vi "demo.vi"() -> ()   [LabVIEW 2014]
uses:
  Instance           7 12Saved   demo .vi
  Instance           3 12Saved   demo .vi
  Instance           6 12Saved   demo .vi
  Instance           4 12Saved   demo .vi
  Instance           5 12Saved   demo .vi
  Instance           2 12Saved   demo .vi
  Instance           1 12Saved   demo .vi
  ControlCAN.dll
panel:
  out "retok1":bool
  out "retok0":bool
  in  "Radio_Baud 2":bool=TRUE
  in  "e-u-baud 2":cluster{"数值":u32}
  out "VCI_INIT_CONFIG 2":T1={"AccCode"=0, "AccMask"=4294967295, "Reserved"=0, "Filter"=1, "Timing0"=0, "Timing1"=20, "Mode"=0}
  in  "?":enum32{"选项卡 1"}(tab)
  out "VF控制频率":dbl caption="Beta"
  out "母线电流":dbl caption="Beta"
  in  "扭矩梯度":dbl caption="Beta"
  in  "打开曲线":bool
  in  "CAN通道0":u32 caption="CAN"
  in  "StartCAN":bool
  in  "设备类型":u32(ring)=1 items=["PCI5121"=1, "PCI9810"=2, "USBCAN1"=3, "USBCAN2"=4, "PCI9820"=5, "PCI5110"=7, "PC104CAN"=11, "CANETUDP"=12, "PCI9840B"=14, "PC104C2"=15, "PCI9820I"=16, "CANETTCP"=17, "PCIE9221"=24, "PCI5010U"=19, "USBCAN_E_U"=20, "USBCAN_2E_U"=21, "PCI5020U"=22, "PCIE9120I"=27, "PCIE9110I"=28, "PCIE9140I"=29]
  in  "OpenDevice":bool
  in  "DeviceOpen":bool
  out "CANStartup":bool
  in  "Baud":u32(ring)=11 caption="波特率" items=["5Kbps", "10Kbps", "20Kbps", "40Kbps", "50Kbps", "80Kbps", "100Kbps", "125Kbps", "200Kbps", "250Kbps", "400Kbps", "500Kbps", "666Kbps", "800Kbps", "1000Kbps"]
  in  "索引":u32(ring) items=["0", "1", "2", "3", "4", "5", "6", "7", "8"]
  out "电位器值":i16 caption="Beta"
  out "母线电流零漂":u16 caption="Beta"
  out "V相电流":dbl
  in  "保存路径 2":path caption="保存路径"
  out "记录计数 3":u32 caption="已记录"
  in  "自动记录 2":bool
  out "U电流零漂":u16 caption="Beta"
  out "V电流零漂":u16 caption="Beta"
  out "U相电流":dbl caption="Beta"
  out "W相电流":dbl caption="Beta"
  in  "控制模式":u8(ring) items=["停车", "速度控制", "扭矩控制"]
  out "母线电压":dbl caption="Beta"
  out "电角度":u16
  out "D轴电压Vd":dbl
  out "Q轴电压Vq":dbl caption="Beta"
  out "Id电流":dbl caption="Beta"
  out "Iq电流":dbl caption="Beta"
  out "Id电流指令":dbl
  out "Iq电流指令":dbl caption="Beta"
  out "控制模式":u8(ring) items=["停车", "速度控制", "扭矩控制", "VqVF控制", "VdVq控制", "IdIq控制"]
  out "相电流Is":dbl caption="Beta"
  out "相电压Vs":dbl caption="Beta"
  in  "确定发送":bool
  in  "转矩指令":dbl caption="Beta"
  out "电机扭矩":dbl caption="Beta"
  in  "转速梯度":dbl caption="Beta"
  in  "增加":bool
  in  "减少":bool
  in  "增加 2":bool
  in  "减少 2":bool
  in  "故障恢复":bool
  out "系统报警码":u16 caption="Beta"
  out "波形图表":T2(graph)
  in  "给定转速":dbl caption="Beta"
  out "电机转速":dbl caption="Beta"
  in  "选项卡控件":enum32{"选项卡 1"}(tab)
  in  "TREvent":T3={"Tx_Or_Rx"=FALSE, "VCI_CAN_OBJ"={"ID"=0, "TimeStamp"=0, "TimeFlag"=0, "SendType"=1, "RemoteFlag"=0, "ExternFlag"=0, "DataLen"=8, 0, 0, 0, 0, 0, 0, 0, 0, 0, 0, 0}, "VCI_CAN_OBJ_N"=[], "Num"=0}
  in  "滤波模式":u32(ring) items=["标准帧滤波", "扩展帧滤波", "禁能滤波"]
  in  "寄存器":u32 format="0x%08x"
  in  "Radio_Baud(E_U)":bool=TRUE
  in  "CANET IP":string
  in  "stop":bool
  in  "发送类型":u8(ring) items=["正常发送", "单次发送", "自发自收", "单次自发自收"]
  in  "帧类型":u8(ring) items=["标准帧", "扩展帧"]
  in  "帧格式":u8(ring) items=["数据帧", "远程帧"]
  in  "数据输入":string
  in  "ID":u32 format="0x%08x"
  in  "验收码":u32 format="0x%08x"
  in  "屏蔽码":u32=4294967295 format="0x%08x"
  in  "BTR0":u8 format="0x%02x"
  in  "BTR1":u8=20 format="0x%02x"
  in  "滤波方式":u8(ring) items=["双滤波", "单滤波"]
  in  "模式":u8(ring) items=["正常", "只听"]
  in  "Clear Buffer":bool
  in  "GetBoardInfo":bool
  in  "GetErrorInfo":bool
  in  "GetStatus":bool
  in  "SEND_NCAN":bool
  in  "滤波结束ID":u32
  in  "滤波起始ID":u32
  in  "一次发送帧数":u32
  in  "Radio_Baud":bool=TRUE
  in  "BTR1 2":u8=20 format="0x%02x"
  in  "BTR0 2":u8 format="0x%02x"
  in  "寄存器 2":u32 format="0x%08x"
  in  "确定发送 2":bool
  in  "ResetCAN":bool
  out "CANStartup 2":bool
  in  "StartCAN 2":bool
  in  "CAN 通道 2":u32=1 caption="CAN"
  in  "Baud 2":u32(ring) caption="波特率2" items=["5Kbps", "10Kbps", "20Kbps", "40Kbps", "50Kbps", "80Kbps", "100Kbps", "125Kbps", "200Kbps", "250Kbps", "400Kbps", "500Kbps", "666Kbps", "800Kbps", "1000Kbps"]
  out "VCI_CAN_OBJ_TN":T4(array[cluster])
  out "VCI_CAN_OBJ_RN":T4(array[cluster])
  in  "arraylen":u32
  out "type":u8[](array[numeric])
  in  "本机端口":u32
  in  "本机类型":enum32{"Radio Selection 1", "Radio Selection 2"}(radio)
  in  "CANET 端口":u32
  out "VCI_FILTER_RECORD":cluster{"ExtFrame":u32, "Start":u32, "End":u32}
  in  "e-u-baud":cluster{"数值":u32}
  out "VCI_CAN_OBJ_T_N":T4(array[cluster])
  out "VCI_BOARD_INFO":T5
  out "VCI_ERR_INFO":T6
  out "VCI_CAN_STATUS":T7
  out "stop 2":bool
  out "Num Rows":u32
  out "TRCount":u32
  out "VCI_CAN_OBJ_R":T8={"ID"=0, "TimeStamp"=0, "TimeFlag"=0, "SendType"=1, "RemoteFlag"=0, "ExternFlag"=0, "DataLen"=8, 0, 0, 0, 0, 0, 0, 0, 0, 0, 0, 0}
  out "VCI_CAN_OBJ_T":T8={"ID"=0, "TimeStamp"=0, "TimeFlag"=0, "SendType"=1, "RemoteFlag"=0, "ExternFlag"=0, "DataLen"=8, 0, 0, 0, 0, 0, 0, 0, 0, 0, 0, 0}
  out "VCI_INIT_CONFIG":T1={"AccCode"=0, "AccMask"=4294967295, "Reserved"=0, "Filter"=1, "Timing0"=0, "Timing1"=20, "Mode"=0}
  # "_U系列特殊设置"
  # "CANET 设备特殊设置"
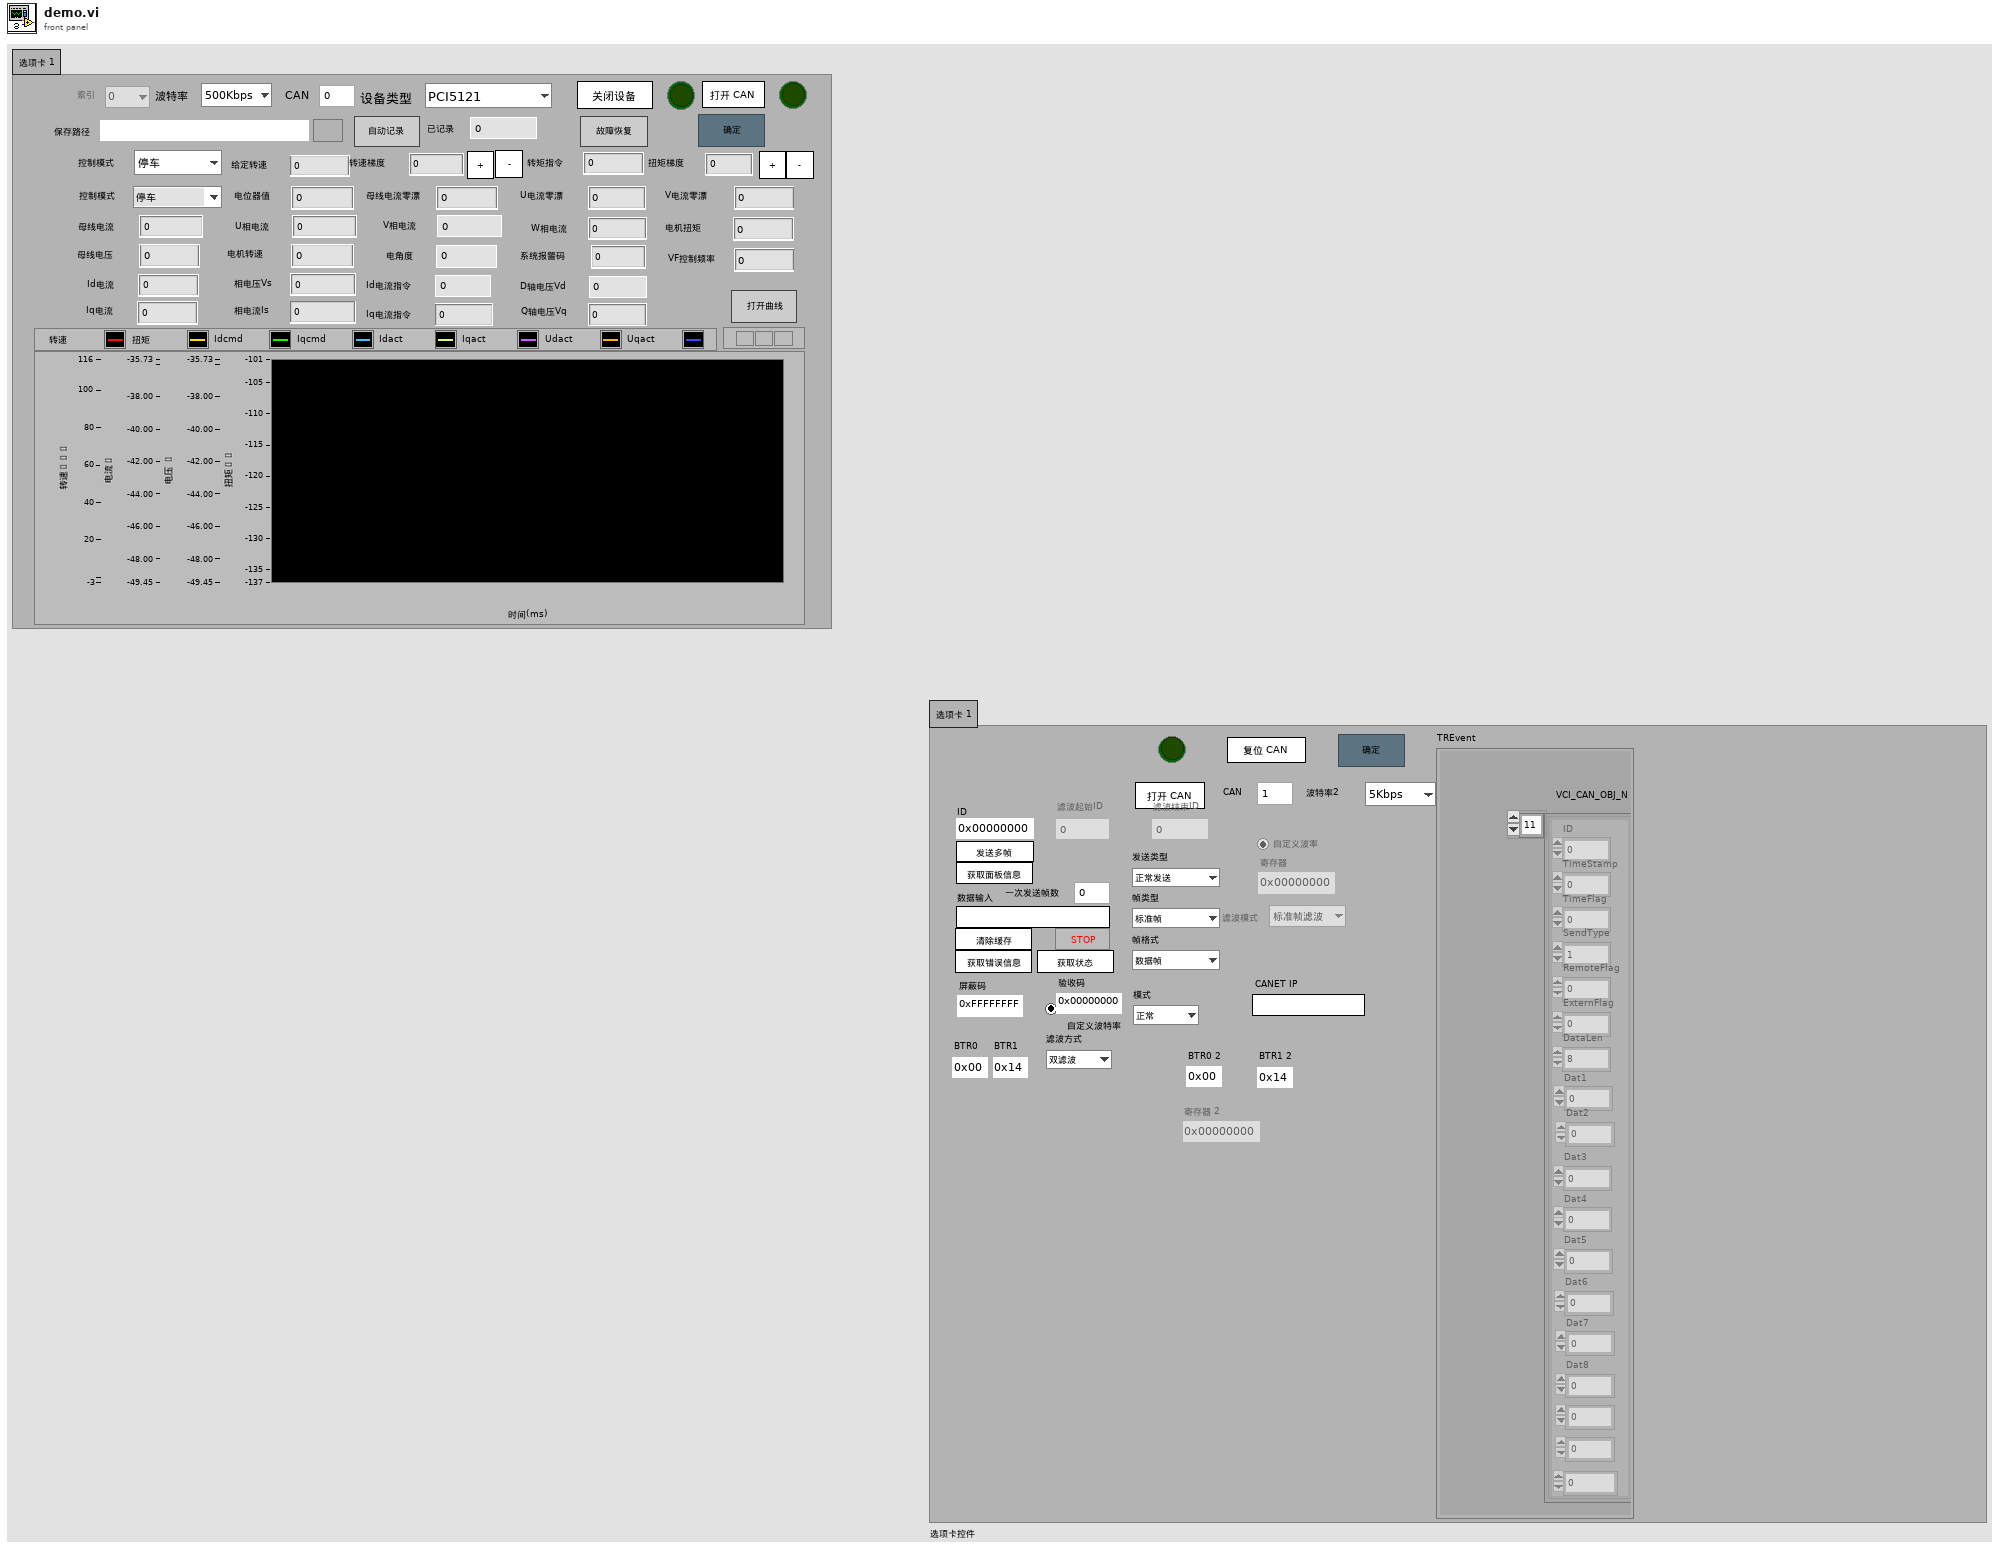
[diagram p1: front panel]
types:
  T1 = cluster{"AccCode":u32, "AccMask":u32, "Reserved":u32, "Filter":u8, "Timing0":u8, "Timing1":u8, "Mode":u8}
  T2 = cluster{"电机转速 ":dbl, " 电机扭矩":dbl, "D轴电流指令":dbl, "Q轴电流指令":dbl, "D轴电流Id":dbl, "Q轴电流Iq":dbl, "D轴电压Vd":dbl, "Q轴电压Vq":dbl}
  T3 = cluster{"Tx_Or_Rx":bool, "VCI_CAN_OBJ":cluster{"ID":u32, "TimeStamp":u32, "TimeFlag":u8, "SendType":u8, "RemoteFlag":u8, "ExternFlag":u8, "DataLen":u8, u8, u8, u8, u8, u8, u8, u8, u8, u8, u8, u8}, "VCI_CAN_OBJ_N":cluster{"ID":u32, "TimeStamp":u32, "TimeFlag":u8, "SendType":u8, "RemoteFlag":u8, "ExternFlag":u8, "DataLen":u8, "Dat1":u8, "Dat2":u8, "Dat3":u8, "Dat4":u8, "Dat5":u8, "Dat6":u8, "Dat7":u8, "Dat8":u8, u8, u8, u8}[], "Num":u32}
  T4 = cluster{"ID":u32, "TimeStamp":u32, "TimeFlag":u8, "SendType":u8, "RemoteFlag":u8, "ExternFlag":u8, "DataLen":u8, u8, u8, u8, u8, u8, u8, u8, u8, u8, u8, u8}[]
  T5 = cluster{"hw_Version":u16, "fw_Version":u16, "dr_Version":u16, "in_Version":u16, "irq_Num":u16, "can_Num":u8, "str_Serial_Num 0":i8, "str_Serial_Num 1":i8, "str_Serial_Num 2":i8, "str_Serial_Num 3":i8, "str_Serial_Num 4":i8, "str_Serial_Num 5":i8, "str_Serial_Num 6":i8, "str_Serial_Num 7":i8, "str_Serial_Num 8":i8, "str_Serial_Num 9":i8, "str_Serial_Num 10":i8, "str_Serial_Num 11":i8, "str_Serial_Num 12":i8, "str_Serial_Num 13":i8, "str_Serial_Num 14":i8, "str_Serial_Num 15":i8, "str_Serial_Num 16":i8, "str_Serial_Num 17":i8, "str_Serial_Num 18":i8, "str_Serial_Num 19":i8, "str_hw_Type 0":i8, "str_hw_Type 1":i8, "str_hw_Type 2":i8, "str_hw_Type 3":i8, "str_hw_Type 4":i8, "str_hw_Type 5":i8, "str_hw_Type 6":i8, "str_hw_Type 7":i8, "str_hw_Type 8":i8, "str_hw_Type 9":i8, "str_hw_Type 10":i8, "str_hw_Type 11":i8, "str_hw_Type 12":i8, "str_hw_Type 13":i8, "str_hw_Type 14":i8, "str_hw_Type 15":i8, "str_hw_Type 16":i8, "str_hw_Type 17":i8, "str_hw_Type 18":i8, "str_hw_Type 19":i8, "str_hw_Type 20":i8, "str_hw_Type 21":i8, "str_hw_Type 22":i8, "str_hw_Type 23":i8, "str_hw_Type 24":i8, "str_hw_Type 25":i8, "str_hw_Type 26":i8, "str_hw_Type 27":i8, "str_hw_Type 28":i8, "str_hw_Type 29":i8, "str_hw_Type 30":i8, "str_hw_Type 31":i8, "str_hw_Type 32":i8, "str_hw_Type 33":i8, "str_hw_Type 34":i8, "str_hw_Type 35":i8, "str_hw_Type 36":i8, "str_hw_Type 37":i8, "str_hw_Type 38":i8, "str_hw_Type 39":i8, "Reserved 0":u16, "Reserved 1":u16, "Reserved 2":u16, "Reserved 3":u16}
  T6 = cluster{"ErrCode":u32, "Passive_ErrData0":u8, "Passive_ErrData1":u8, "Passive_ErrData2":u8, "ArLost_ErrData":u8}
  T7 = cluster{"ErrInterrupt":u8, "regMode":u8, "regStatus":u8, "regALCapture":u8, "regECCapture":u8, "regEWLimit":u8, "regRECounter":u8, "regTECounter":u8, "Reserved":u32}
  T8 = cluster{"ID":u32, "TimeStamp":u32, "TimeFlag":u8, "SendType":u8, "RemoteFlag":u8, "ExternFlag":u8, "DataLen":u8, u8, u8, u8, u8, u8, u8, u8, u8, u8, u8, u8}
  T9 = cluster{"[0]":u32, "[1]":u32, "[2]":u32, "[3]":u32, "[4]":u32, "[5]":u32, "[6]":u32, "[7]":u32, "[8]":u32}
  T10 = cluster{"ID":u32, u32, u8, "发送类型":u8, "帧格式":u8, "帧类型":u8, i32, "[0]":u32, "[1]":u32, "[2]":u32, "[3]":u32, "[4]":u32, "[5]":u32, "[6]":u32, "[7]":u32, u8, u8, u8}
  T11 = cluster{"验收码":u32, "屏蔽码":u32, i32, "滤波方式":u8, "BTR0 2":u8, "BTR1 2":u8, "模式":u8}
  T12 = cluster{"验收码":u32, "屏蔽码":u32, u32, "滤波方式":u8, "BTR0":u8, "BTR1":u8, "模式":u8}
  T13 = cluster{"ID":u32, "TimeStamp":u32, "TimeFlag":u8, "SendType":u8, "RemoteFlag":u8, "ExternFlag":u8, "DataLen":u8, "Dat1":u8, "Dat2":u8, "Dat3":u8, "Dat4":u8, "Dat5":u8, "Dat6":u8, "Dat7":u8, "Dat8":u8, u8, u8, u8}[]
  T14 = cluster{"0x55":u32, u32, u8, "发送类型":u8, "帧格式":u8, "帧类型":u8, i32, "控制模式":u8, i16, u8, u8, u8, u8, u8, u8, u8, u8, u8}
  T15 = cluster{"0x55":u32, u32, u8, "发送类型":u8, "帧格式":u8, "帧类型":u8, i32, "控制模式":u8, u8, u8, u8, u8, u8, u8, u8, u8, u8, u8}
  T16 = cluster{bool, "VCI_CAN_OBJ_R":cluster{"ID":u32, "TimeStamp":u32, "TimeFlag":u8, "SendType":u8, "RemoteFlag":u8, "ExternFlag":u8, "DataLen":u8, u8, u8, u8, u8, u8, u8, u8, u8, u8, u8, u8}, "pReceive":cluster{"ID":u32, "TimeStamp":u32, "TimeFlag":u8, "SendType":u8, "RemoteFlag":u8, "ExternFlag":u8, "DataLen":u8, u8, u8, u8, u8, u8, u8, u8, u8, u8, u8, u8}[], "return type":u32}
  T17 = cluster{bool, "VCI_CAN_OBJ_T":cluster{"ID":u32, "TimeStamp":u32, "TimeFlag":u8, "SendType":u8, "RemoteFlag":u8, "ExternFlag":u8, "DataLen":u8, u8, u8, u8, u8, u8, u8, u8, u8, u8, u8, u8}, cluster{"ID":u32, "TimeStamp":u32, "TimeFlag":u8, "SendType":u8, "RemoteFlag":u8, "ExternFlag":u8, "DataLen":u8, u8, u8, u8, u8, u8, u8, u8, u8, u8, u8, u8}[], "return type":u32}
  T18 = cluster{"电机转速 ":dbl, " 电机扭矩":dbl, "Id电流指令":dbl, "Iq电流指令":dbl, "Id电流":dbl, "Iq电流":dbl, "D轴电压Vd":dbl, "Q轴电压Vq":dbl}
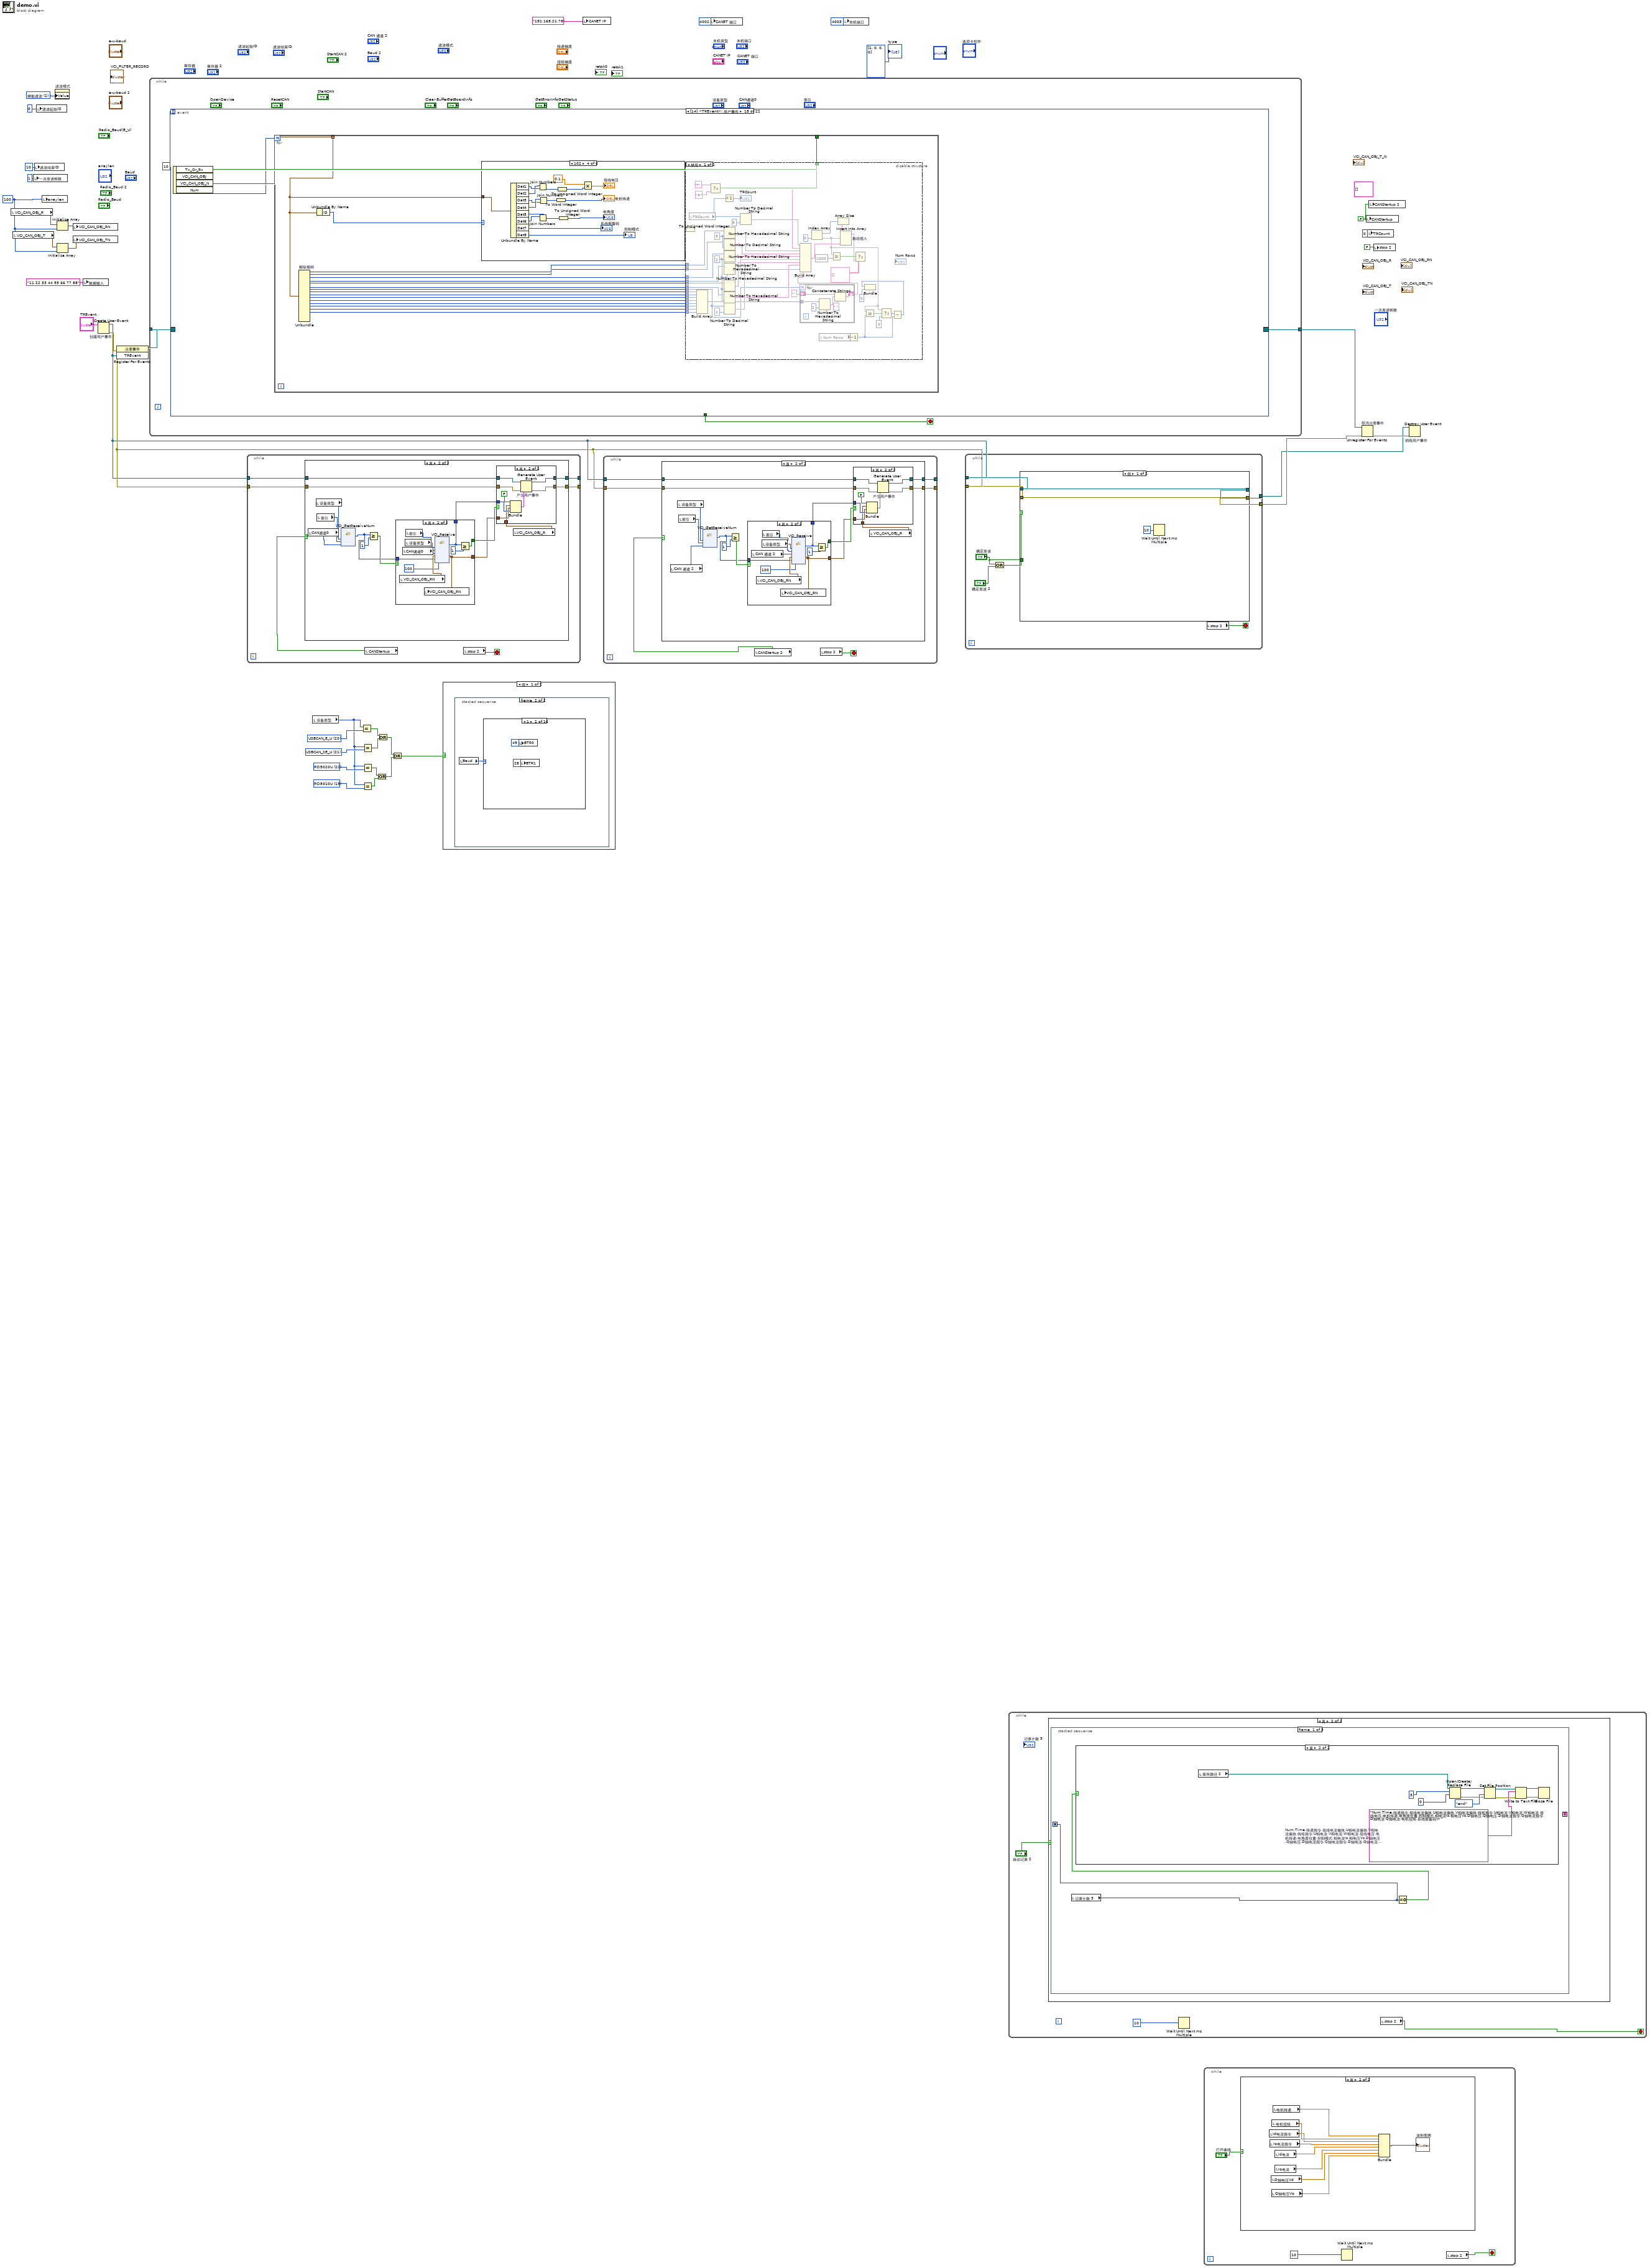
[diagram p0: block diagram]
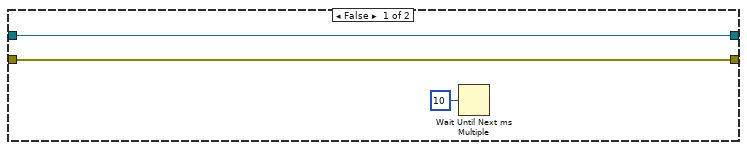
[diagram p2: hidden frame]
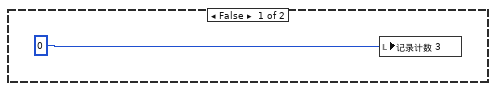
[diagram p6: hidden frame]
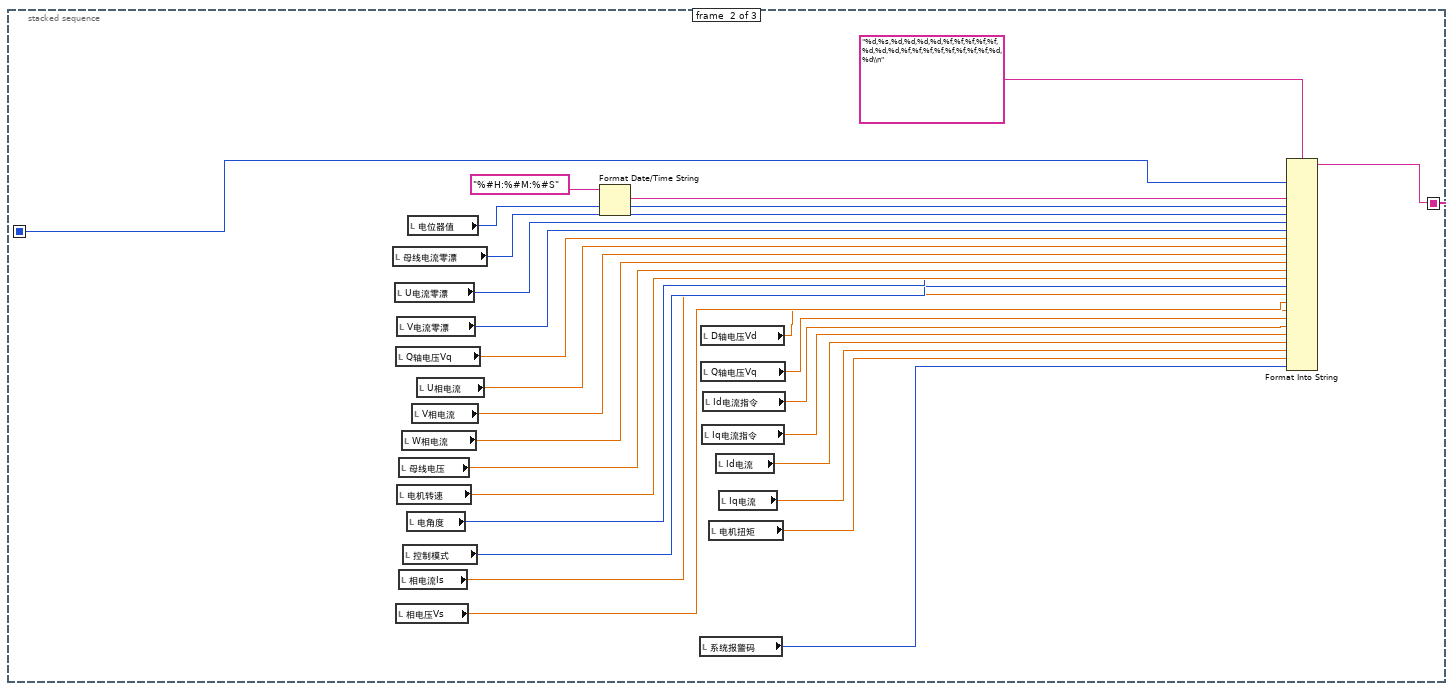
[diagram p8: hidden frame]
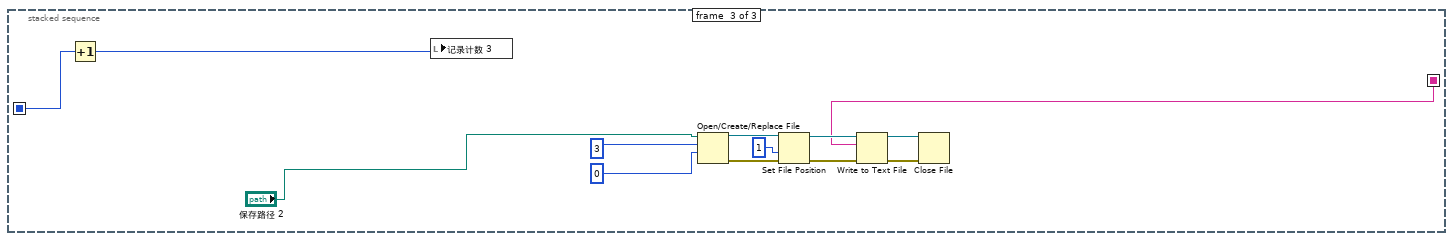
[diagram p9: hidden frame]
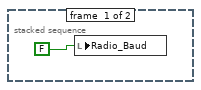
[diagram p10: hidden frame]
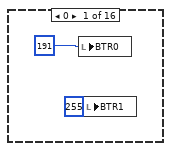
[diagram p11: hidden frame]
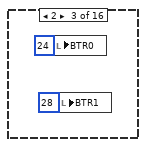
[diagram p12: hidden frame]
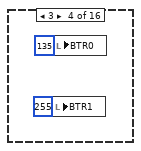
[diagram p13: hidden frame]
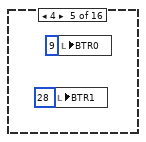
[diagram p14: hidden frame]
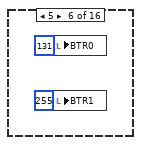
[diagram p15: hidden frame]
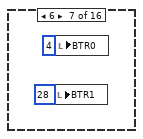
[diagram p16: hidden frame]
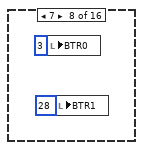
[diagram p17: hidden frame]
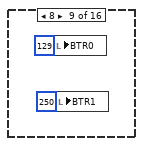
[diagram p18: hidden frame]
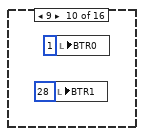
[diagram p19: hidden frame]
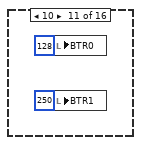
[diagram p20: hidden frame]
diagram:
  w13 = u32 19 items=["PCI5121"=1, "PCI9810"=2, "USBCAN1"=3, "USBCAN2"=4, "PCI9820"=5, "PCI5110"=7, "CANLite(mini)"=8, "ISA9620"=9, "ISA5420"=10, "PC104CAN"=11, "DNP9810"=13, "PCI9840B"=14, "PC104C2"=15, "PCI9820I"=16, "pec9920"=18, "PCI5010U"=19, "USBCAN_E_U"=20, "USBCAN_2E_U"=21, "PCI5020U"=22, ""=0] ("DeviceType")
  w14 = u32 22 items=["PCI5121"=1, "PCI9810"=2, "USBCAN1"=3, "USBCAN2"=4, "PCI9820"=5, "PCI5110"=7, "CANLite(mini)"=8, "ISA9620"=9, "ISA5420"=10, "PC104CAN"=11, "DNP9810"=13, "PCI9840B"=14, "PC104C2"=15, "PCI9820I"=16, "pec9920"=18, "PCI5010U"=19, "USBCAN_E_U"=20, "USBCAN_2E_U"=21, "PCI5020U"=22, ""=0] ("DeviceType")
  w15 = u32 21 items=["PCI5121"=1, "PCI9810"=2, "USBCAN1"=3, "USBCAN2"=4, "PCI9820"=5, "PCI5110"=7, "CANLite(mini)"=8, "ISA9620"=9, "ISA5420"=10, "PC104CAN"=11, "DNP9810"=13, "PCI9840B"=14, "PC104C2"=15, "PCI9820I"=16, "pec9920"=18, "USBCAN_E_U"=20, "USBCAN_2E_U"=21, ""=0] ("DeviceType")
  w16 = u32 20 items=["PCI5121"=1, "PCI9810"=2, "USBCAN1"=3, "USBCAN2"=4, "PCI9820"=5, "PCI5110"=7, "CANLite(mini)"=8, "ISA9620"=9, "ISA5420"=10, "PC104CAN"=11, "DNP9810"=13, "PCI9840B"=14, "PC104C2"=15, "PCI9820I"=16, "pec9920"=18, "USBCAN_E_U"=20, "USBCAN_2E_U"=21, ""=0] ("DeviceType")
  w22 = u32 100 ("arraylen")
  w30 = u32 2 items=["标准帧滤波", "扩展帧滤波", "禁能滤波"] ("fiter_mode")
  (unwired) string[][] [] ("Item Names")
  w4 = FALSE
  n1 = local read "VCI_CAN_OBJ_R"() -> (w25:T8)
  n2 = local read "VCI_CAN_OBJ_T"() -> (w23:T8)
  n3 = local write "一次发送帧数"(u32 1 ("一次发送帧数")) -> ()
  n4 = local write "滤波结束ID"(u32 10 ("fiter_endid")) -> ()
  n5 = local write "滤波起始ID"(u32 0 ("fiter_startid")) -> ()
  n6 = local write "arraylen"(w22) -> ()
  n7 = property on="滤波模式" class="Ring (严格)"("Value"=w30) -> ()  [unwired: 2 in, 2 out]
  n8 = Initialize Array(w25, w22) -> (w24:T4)
  n9 = Initialize Array(w23, w22) -> (w21:T4)
  n10 = local write "VCI_CAN_OBJ_RN"(w24) -> ()
  n11 = local write "VCI_CAN_OBJ_TN"(w21) -> ()
  n12 = local write "数据输入"("11 22 33 44 55 66 77 88" ("Data Input")) -> ()
  n13 = Create User Event "创建用户事件"(user event datatype="TREvent") -> (user event=w3:refnum<user-event>, error out=w37:errorcluster)  [unwired: 1 in]
  n14 = register-events(error in=w37, w3) -> (reference out=w34:refnum<event-registration>, error out=w2:errorcluster)  [unwired: 1 in]
  n15 = while {
    tunnel: w34 -> [w42]
    tunnel: [w41] -> w1
    stop <- w39 stop-if-true
    n16 = event shown="[14] <TREvent>: 用户事件" {
      selector: w42 -> [_ _ _ _ _ _ _ _ _ _ _ _ _ _ _ _ _ _ _ _ _ _]
      dyn-events: [_ _ _ _ _ _ _ _ _ _ _ _ _ _ _ _ _ _ _ _ _ _] -> w41
      timeout: 10 -> [_ _ _ _ _ _ _ _ _ _ _ _ _ _ _ _ _ _ _ _ _ _]
      tunnel: [_ _ _ _ w300 _ _ _ _ _ _ _ _ _ _ _ _ _ _ _ _ _] -> w39
      event Timeout {
        n17 = event-data() -> ()  [unwired: 2 out]
        n18 = local read "滤波结束ID"() -> (w61:u32)
        n19 = local read "滤波起始ID"() -> (w62:u32)
        n20 = local read "滤波模式"() -> (w64:u32)
        n21 = local read "CAN通道0"() -> (w66:u32)
        n22 = local read "设备类型"() -> (w55:u32)
        n23 = local read "索引"() -> (w54:u32)
        n24 = local read "CAN 通道 2"() -> (w53:u32)
        n25 = Bundle("滤波模式"=w64, "滤波起始ID"=w62, "滤波结束ID"=w61) -> (w63:cluster{"滤波模式":u32, "滤波起始ID":u32, "滤波结束ID":u32})  [unwired: 1 out]
        n26 = dll-call lib="PTH2Kabs J2车用永磁同步电机测试上位机CAN2_源码ControlCAN.dll" fn="VCI_GetReceiveNum"("DeviceType"=w55, "DeviceInd"=w54, "CANInd"=w66) -> ()  [unwired: 6 in, 3 out]
        n27 = dll-call lib="PTH2Kabs J2车用永磁同步电机测试上位机CAN2_源码ControlCAN.dll" fn="VCI_GetReceiveNum"("DeviceType"=w55, "DeviceInd"=w54, "CANInd"=w53) -> ()  [unwired: 6 in, 3 out]
        n28 = disable-structure shown="禁用" {
          disable-tunnel: "帧格式" -> [w80 _]
          disable-tunnel: "帧类型" -> [w79 _]
          disable-tunnel: "发送类型" -> [w78 _]
          disable-tunnel: "ID" -> [w71 _]
          frame Disabled {
            w89 = u8 0
            w77 = u32 0
            n29 = for {
              N: 8 -> [_]
              tunnel: "数据输入" -> [w104]
              tunnel: [w107] -> w75 mode=indexing
              tunnel: [w92] -> w73
              i -> [w97]
              n30 = Multiply(x=3, y=w97) -> (x*y=w110:i32)
              n31 = String Length(string=w104) -> (length=w103:i32)
              n32 = String Subset(string=w104, offset (0)=w110, length (rest)=2 ("length (rest)")) -> (substring=w101:string)
              n33 = Quotient & Remainder(x=w103, y=3) -> (x-y*floor(x/y)=w99:i32, floor(x/y)=w95:i32)
              n34 = Equal To 0?(x=w99) -> (x = 0?=w98:bool)
              n35 = Increment(x=w95) -> (x+1=w96:i32)
              n36 = Hex Digit?(1:w101) -> (0:w105:bool)
              n37 = Select(t=w95, s=w98, f=w96) -> (s? t:f=w94:i32)
              n38 = Select(t=w101, s=w105, f="00" ("t")) -> (s? t:f=w106:string)
              n39 = Quotient & Remainder(x=w94, y=9) -> (x-y*floor(x/y)=w92:i32)  [unwired: 1 out]
              n40 = Scan From String(format string="%2x ", input string=w106) -> (output 1=w107:u32)  [unwired: 2 in, 4 out]
            }
            n41 = Array To Cluster(array=w75) -> (cluster=w74:T9)
            n42 = Unbundle(w74) -> ("[0]"=w81:u32, "[1]"=w82:u32, "[2]"=w83:u32, "[3]"=w84:u32, "[4]"=w85:u32, "[5]"=w86:u32, "[6]"=w87:u32, "[7]"=w88:u32)  [unwired: 1 out]
            n43 = To Unsigned Byte Integer(number=w77) -> (unsigned 8bit integer=w76:u8)
            n44 = Bundle("ID"=w71, w77, w76, "发送类型"=w78, "帧格式"=w80, "帧类型"=w79, w73, "[0]"=w81, "[1]"=w82, "[2]"=w83, "[3]"=w84, "[4]"=w85, "[5]"=w86, "[6]"=w87, "[7]"=w88, w89, w89, w89) -> (w91:T10)  [unwired: 1 out]
            n45 = local write "VCI_CAN_OBJ_T"(w91) -> ()
          }
          frame Enabled {
          }
        }
        n46 = local write "VCI_FILTER_RECORD"(w63) -> ()
        n47 = Bundle("验收码"="验收码", "屏蔽码"="屏蔽码", 0, "滤波方式"="滤波方式", "BTR0 2"="BTR0 2", "BTR1 2"="BTR1 2", "模式"="模式") -> (→"VCI_INIT_CONFIG 2":T11)  [unwired: 1 out]
        n48 = Bundle("验收码"="验收码", "屏蔽码"="屏蔽码", u32 0, "滤波方式"="滤波方式", "BTR0"="BTR0", "BTR1"="BTR1", "模式"="模式") -> (→"VCI_INIT_CONFIG":T12)  [unwired: 1 out]
        n49 = local read "寄存器 2"() -> (w43:u32)
        n50 = local read "寄存器"() -> (w60:u32)
        n51 = Bundle("寄存器 2"=w43) -> (w44:cluster{"寄存器 2":u32})  [unwired: 1 in]
        n52 = Bundle("寄存器"=w60) -> (w65:cluster{"寄存器":u32})  [unwired: 1 in]
        n53 = local write "e-u-baud"(w65) -> ()
        n54 = local write "e-u-baud 2"(w44) -> ()
      }
      event "Baud": Value Change {
        w120 = u32 19 items=["PCI5121"=1, "PCI9810"=2, "USBCAN1"=3, "USBCAN2"=4, "PCI9820"=5, "PCI5110"=7, "CANLite(mini)"=8, "ISA9620"=9, "ISA5420"=10, "PC104CAN"=11, "DNP9810"=13, "PCI9840B"=14, "PC104C2"=15, "PCI9820I"=16, "pec9920"=18, "PCI5010U"=19, "USBCAN_E_U"=20, "USBCAN_2E_U"=21, "PCI5020U"=22, ""=0] ("DeviceType")
        w121 = u32 22 items=["PCI5121"=1, "PCI9810"=2, "USBCAN1"=3, "USBCAN2"=4, "PCI9820"=5, "PCI5110"=7, "CANLite(mini)"=8, "ISA9620"=9, "ISA5420"=10, "PC104CAN"=11, "DNP9810"=13, "PCI9840B"=14, "PC104C2"=15, "PCI9820I"=16, "pec9920"=18, "PCI5010U"=19, "USBCAN_E_U"=20, "USBCAN_2E_U"=21, "PCI5020U"=22, ""=0] ("DeviceType")
        w122 = u32 21 items=["PCI5121"=1, "PCI9810"=2, "USBCAN1"=3, "USBCAN2"=4, "PCI9820"=5, "PCI5110"=7, "CANLite(mini)"=8, "ISA9620"=9, "ISA5420"=10, "PC104CAN"=11, "DNP9810"=13, "PCI9840B"=14, "PC104C2"=15, "PCI9820I"=16, "pec9920"=18, "USBCAN_E_U"=20, "USBCAN_2E_U"=21, ""=0] ("DeviceType")
        w123 = u32 20 items=["PCI5121"=1, "PCI9810"=2, "USBCAN1"=3, "USBCAN2"=4, "PCI9820"=5, "PCI5110"=7, "CANLite(mini)"=8, "ISA9620"=9, "ISA5420"=10, "PC104CAN"=11, "DNP9810"=13, "PCI9840B"=14, "PC104C2"=15, "PCI9820I"=16, "pec9920"=18, "USBCAN_E_U"=20, "USBCAN_2E_U"=21, ""=0] ("DeviceType")
        n55 = event-data() -> ()  [unwired: 7 out]
        n56 = local read "设备类型"() -> (w119:u32)
        n57 = local read "Baud"() -> (w124:u32)
        n58 = Equal?(x=w119, y=w123) -> (x = y?=w118:bool)
        n59 = Equal?(x=w119, y=w122) -> (x = y?=w117:bool)
        n60 = Equal?(x=w119, y=w121) -> (x = y?=w116:bool)
        n61 = Equal?(x=w119, y=w120) -> (x = y?=w115:bool)
        n62 = Or(x=w116, y=w115) -> (x .or. y?=w113:bool)
        n63 = Or(x=w118, y=w117) -> (x .or. y?=w114:bool)
        n64 = Or(x=w114, y=w113) -> (x .or. y?=w112:bool)
        n65 = case shown="14" w124 {
          frame 0 {
            n66 = local write "BTR0"(u8 191 ("BTR0")) -> ()
            n67 = local write "BTR1"(u8 255 ("BTR1")) -> ()
          }
          frame 1 {
            n68 = local write "BTR0"(49) -> ()
            n69 = local write "BTR1"(28) -> ()
          }
          frame 2 {
            n70 = local write "BTR0"(24) -> ()
            n71 = local write "BTR1"(28) -> ()
          }
          frame 3 {
            n72 = local write "BTR0"(135) -> ()
            n73 = local write "BTR1"(255) -> ()
          }
          frame 4 {
            n74 = local write "BTR0"(9) -> ()
            n75 = local write "BTR1"(28) -> ()
          }
          frame 5 {
            n76 = local write "BTR1"(255) -> ()
            n77 = local write "BTR0"(131) -> ()
          }
          frame 6 {
            n78 = local write "BTR1"(28) -> ()
            n79 = local write "BTR0"(4) -> ()
          }
          frame 7 {
            n80 = local write "BTR1"(28) -> ()
            n81 = local write "BTR0"(3) -> ()
          }
          frame 8 {
            n82 = local write "BTR0"(129) -> ()
            n83 = local write "BTR1"(250) -> ()
          }
          frame 9 {
            n84 = local write "BTR0"(1) -> ()
            n85 = local write "BTR1"(28) -> ()
          }
          frame 10 {
            n86 = local write "BTR1"(250) -> ()
            n87 = local write "BTR0"(128) -> ()
          }
          frame 11 {
            n88 = local write "BTR0"(0) -> ()
            n89 = local write "BTR1"(28) -> ()
          }
          frame 12 {
            n90 = local write "BTR1"(182) -> ()
            n91 = local write "BTR0"(128) -> ()
          }
          frame 13 {
            n92 = local write "BTR0"(0) -> ()
            n93 = local write "BTR1"(22) -> ()
          }
          frame 14 {
            n94 = local write "BTR0"(0) -> ()
            n95 = local write "BTR1"(20) -> ()
          }
          frame 15, Default {
            n96 = local write "BTR0"(1) -> ()
            n97 = local write "BTR1"(1) -> ()
          }
        }
        n98 = case shown="假" w112 {
          frame False {
            n99 = stacked-sequence {
              frame #0 {
                n100 = local write "Radio_Baud"(FALSE) -> ()
              }
              frame #1 {
                n101 = local read "Baud"() -> (w126:u32)
                n102 = case shown="7" w126 {
                  frame 0 {
                    n103 = local write "BTR0"(u8 191 ("BTR0")) -> ()
                    n104 = local write "BTR1"(u8 255 ("BTR1")) -> ()
                  }
                  frame 1 {
                    n105 = local write "BTR0"(u8 49 ("BTR0")) -> ()
                    n106 = local write "BTR1"(u8 28 ("BTR1")) -> ()
                  }
                  frame 2 {
                    n107 = local write "BTR0"(u8 24 ("BTR0")) -> ()
                    n108 = local write "BTR1"(u8 28 ("BTR1")) -> ()
                  }
                  frame 3 {
                    n109 = local write "BTR1"(u8 255 ("BTR1")) -> ()
                    n110 = local write "BTR0"(u8 135 ("BTR0")) -> ()
                  }
                  frame 4 {
                    n111 = local write "BTR1"(u8 28 ("BTR1")) -> ()
                    n112 = local write "BTR0"(u8 9 ("BTR0")) -> ()
                  }
                  frame 5 {
                    n113 = local write "BTR0"(u8 131 ("BTR0")) -> ()
                    n114 = local write "BTR1"(u8 255 ("BTR1")) -> ()
                  }
                  frame 6 {
                    n115 = local write "BTR1"(u8 28 ("BTR1")) -> ()
                    n116 = local write "BTR0"(u8 4 ("BTR0")) -> ()
                  }
                  frame 7 {
                    n117 = local write "BTR0"(u8 3 ("BTR0")) -> ()
                    n118 = local write "BTR1"(u8 28 ("BTR1")) -> ()
                  }
                  frame 8 {
                    n119 = local write "BTR0"(u8 129 ("BTR0")) -> ()
                    n120 = local write "BTR1"(u8 250 ("BTR1")) -> ()
                  }
                  frame 9 {
                    n121 = local write "BTR1"(u8 28 ("BTR1")) -> ()
                    n122 = local write "BTR0"(u8 1 ("BTR0")) -> ()
                  }
                  frame 10 {
                    n123 = local write "BTR0"(u8 128 ("BTR0")) -> ()
                    n124 = local write "BTR1"(u8 250 ("BTR1")) -> ()
                  }
                  frame 11 {
                    n125 = local write "BTR0"(u8 0 ("BTR0")) -> ()
                    n126 = local write "BTR1"(u8 28 ("BTR1")) -> ()
                  }
                  frame 12 {
                    n127 = local write "BTR0"(u8 128 ("BTR0")) -> ()
                    n128 = local write "BTR1"(u8 182 ("BTR1")) -> ()
                  }
                  frame 13 {
                    n129 = local write "BTR1"(u8 22 ("BTR1")) -> ()
                    n130 = local write "BTR0"(u8 0 ("BTR0")) -> ()
                  }
                  frame 14 {
                    n131 = local write "BTR0"(u8 0 ("BTR0")) -> ()
                    n132 = local write "BTR1"(u8 20 ("BTR1")) -> ()
                  }
                  frame 15, Default {
                  }
                }
              }
            }
          }
          frame True {
            n133 = stacked-sequence {
              frame #0 {
                n134 = local write "Radio_Baud(E_U)"(FALSE) -> ()
                n135 = local write "BTR1"(u8 0 ("BTR1")) -> ()
                n136 = local write "BTR0"(u8 0 ("BTR0")) -> ()
              }
              frame #1 {
                n137 = local read "Baud"() -> (w160:u32)
                n138 = case shown="15, 默认" w160 {
                  frame 15, Default {
                  }
                  frame 14 {
                    n139 = local write "寄存器"(393219) -> ()
                  }
                  frame 13 {
                    n140 = local write "寄存器"(393220) -> ()
                  }
                  frame 11 {
                    n141 = local write "寄存器"(393223) -> ()
                  }
                  frame 9 {
                    n142 = local write "寄存器"(1835016) -> ()
                  }
                  frame 7 {
                    n143 = local write "寄存器"(1835025) -> ()
                  }
                  frame 6 {
                    n144 = local write "寄存器"(1441827) -> ()
                  }
                  frame 4 {
                    n145 = local write "寄存器"(1835052) -> ()
                  }
                  frame 2 {
                    n146 = local write "寄存器"(1441971) -> ()
                  }
                  frame 1 {
                    n147 = local write "寄存器"(1835232) -> ()
                  }
                  frame 0 {
                    n148 = local write "寄存器"(1835457) -> ()
                  }
                }
              }
            }
          }
        }
      }
      event "Baud 2": Value Change {
        w212 = u32 19 items=["PCI5121"=1, "PCI9810"=2, "USBCAN1"=3, "USBCAN2"=4, "PCI9820"=5, "PCI5110"=7, "CANLite(mini)"=8, "ISA9620"=9, "ISA5420"=10, "PC104CAN"=11, "DNP9810"=13, "PCI9840B"=14, "PC104C2"=15, "PCI9820I"=16, "pec9920"=18, "PCI5010U"=19, "USBCAN_E_U"=20, "USBCAN_2E_U"=21, "PCI5020U"=22, ""=0] ("DeviceType")
        w213 = u32 22 items=["PCI5121"=1, "PCI9810"=2, "USBCAN1"=3, "USBCAN2"=4, "PCI9820"=5, "PCI5110"=7, "CANLite(mini)"=8, "ISA9620"=9, "ISA5420"=10, "PC104CAN"=11, "DNP9810"=13, "PCI9840B"=14, "PC104C2"=15, "PCI9820I"=16, "pec9920"=18, "PCI5010U"=19, "USBCAN_E_U"=20, "USBCAN_2E_U"=21, "PCI5020U"=22, ""=0] ("DeviceType")
        w214 = u32 21 items=["PCI5121"=1, "PCI9810"=2, "USBCAN1"=3, "USBCAN2"=4, "PCI9820"=5, "PCI5110"=7, "CANLite(mini)"=8, "ISA9620"=9, "ISA5420"=10, "PC104CAN"=11, "DNP9810"=13, "PCI9840B"=14, "PC104C2"=15, "PCI9820I"=16, "pec9920"=18, "USBCAN_E_U"=20, "USBCAN_2E_U"=21, ""=0] ("DeviceType")
        w215 = u32 20 items=["PCI5121"=1, "PCI9810"=2, "USBCAN1"=3, "USBCAN2"=4, "PCI9820"=5, "PCI5110"=7, "CANLite(mini)"=8, "ISA9620"=9, "ISA5420"=10, "PC104CAN"=11, "DNP9810"=13, "PCI9840B"=14, "PC104C2"=15, "PCI9820I"=16, "pec9920"=18, "USBCAN_E_U"=20, "USBCAN_2E_U"=21, ""=0] ("DeviceType")
        n149 = event-data() -> ()  [unwired: 7 out]
        n150 = local read "设备类型"() -> (w211:u32)
        n151 = Equal?(x=w211, y=w215) -> (x = y?=w210:bool)
        n152 = Equal?(x=w211, y=w214) -> (x = y?=w209:bool)
        n153 = Equal?(x=w211, y=w213) -> (x = y?=w208:bool)
        n154 = Equal?(x=w211, y=w212) -> (x = y?=w207:bool)
        n155 = Or(x=w208, y=w207) -> (x .or. y?=w205:bool)
        n156 = Or(x=w210, y=w209) -> (x .or. y?=w206:bool)
        n157 = Or(x=w206, y=w205) -> (x .or. y?=w204:bool)
        n158 = local read "Baud 2"() -> (w203:u32)
        n159 = case shown="真" w204 {
          frame False {
            n160 = stacked-sequence {
              frame #0 {
                n161 = local write "Radio_Baud 2"(FALSE) -> ()
              }
              frame #1 {
                n162 = local read "Baud 2"() -> (w217:u32)
                n163 = case shown="0" w217 {
                  frame 0 {
                    n164 = local write "BTR0 2"(u8 191 ("BTR0")) -> ()
                    n165 = local write "BTR1 2"(u8 255 ("BTR1")) -> ()
                  }
                  frame 1 {
                    n166 = local write "BTR0 2"(u8 49 ("BTR0")) -> ()
                    n167 = local write "BTR1 2"(u8 28 ("BTR1")) -> ()
                  }
                  frame 2 {
                    n168 = local write "BTR0 2"(u8 24 ("BTR0")) -> ()
                    n169 = local write "BTR1 2"(u8 28 ("BTR1")) -> ()
                  }
                  frame 3 {
                    n170 = local write "BTR0 2"(u8 135 ("BTR0")) -> ()
                    n171 = local write "BTR1 2"(u8 255 ("BTR1")) -> ()
                  }
                  frame 4 {
                    n172 = local write "BTR0 2"(u8 9 ("BTR0")) -> ()
                    n173 = local write "BTR1 2"(u8 28 ("BTR1")) -> ()
                  }
                  frame 5 {
                    n174 = local write "BTR0 2"(u8 131 ("BTR0")) -> ()
                    n175 = local write "BTR1 2"(u8 255 ("BTR1")) -> ()
                  }
                  frame 6 {
                    n176 = local write "BTR0 2"(u8 4 ("BTR0")) -> ()
                    n177 = local write "BTR1 2"(u8 28 ("BTR1")) -> ()
                  }
                  frame 7 {
                    n178 = local write "BTR0 2"(u8 3 ("BTR0")) -> ()
                    n179 = local write "BTR1 2"(u8 28 ("BTR1")) -> ()
                  }
                  frame 8 {
                    n180 = local write "BTR0 2"(u8 129 ("BTR0")) -> ()
                    n181 = local write "BTR1 2"(u8 250 ("BTR1")) -> ()
                  }
                  frame 9 {
                    n182 = local write "BTR0 2"(u8 1 ("BTR0")) -> ()
                    n183 = local write "BTR1 2"(u8 28 ("BTR1")) -> ()
                  }
                  frame 10 {
                    n184 = local write "BTR0 2"(u8 128 ("BTR0")) -> ()
                    n185 = local write "BTR1 2"(u8 250 ("BTR1")) -> ()
                  }
                  frame 11 {
                    n186 = local write "BTR0 2"(u8 0 ("BTR0")) -> ()
                    n187 = local write "BTR1 2"(u8 28 ("BTR1")) -> ()
                  }
                  frame 12 {
                    n188 = local write "BTR0 2"(u8 128 ("BTR0")) -> ()
                    n189 = local write "BTR1 2"(u8 182 ("BTR1")) -> ()
                  }
                  frame 13 {
                    n190 = local write "BTR0 2"(u8 0 ("BTR0")) -> ()
                    n191 = local write "BTR1 2"(u8 22 ("BTR1")) -> ()
                  }
                  frame 14 {
                    n192 = local write "BTR0 2"(u8 0 ("BTR0")) -> ()
                    n193 = local write "BTR1 2"(u8 20 ("BTR1")) -> ()
                  }
                  frame 15, Default {
                  }
                }
              }
            }
          }
          frame True {
            n194 = stacked-sequence {
              frame #0 {
                w248 = u8 0 ("BTR1")
                n195 = local write "Radio_Baud(E_U)"(FALSE) -> ()
                n196 = local write "BTR0 2"(w248) -> ()
                n197 = local write "BTR1 2"(w248) -> ()
              }
              frame #1 {
                n198 = local read "Baud 2"() -> (w250:u32)
                n199 = case shown="14" w250 {
                  frame 15, Default {
                  }
                  frame 14 {
                    n200 = local write "寄存器 2"(393219) -> ()
                  }
                  frame 13 {
                    n201 = local write "寄存器 2"(393220) -> ()
                  }
                  frame 11 {
                    n202 = local write "寄存器 2"(393223) -> ()
                  }
                  frame 9 {
                    n203 = local write "寄存器 2"(1835016) -> ()
                  }
                  frame 7 {
                    n204 = local write "寄存器 2"(1835025) -> ()
                  }
                  frame 6 {
                    n205 = local write "寄存器 2"(1441827) -> ()
                  }
                  frame 4 {
                    n206 = local write "寄存器 2"(1835052) -> ()
                  }
                  frame 2 {
                    n207 = local write "寄存器 2"(1441971) -> ()
                  }
                  frame 1 {
                    n208 = local write "寄存器 2"(1835232) -> ()
                  }
                  frame 0 {
                    n209 = local write "寄存器 2"(1835457) -> ()
                  }
                }
              }
            }
          }
        }
        n210 = case shown="0" w203 {
          frame 0 {
            n211 = local write "BTR0 2"(u8 191 ("BTR0")) -> ()
            n212 = local write "BTR1 2"(u8 255 ("BTR1")) -> ()
          }
          frame 1 {
            n213 = local write "BTR0 2"(49) -> ()
            n214 = local write "BTR1 2"(28) -> ()
          }
          frame 2 {
            n215 = local write "BTR0 2"(24) -> ()
            n216 = local write "BTR1 2"(28) -> ()
          }
          frame 3 {
            n217 = local write "BTR0 2"(135) -> ()
            n218 = local write "BTR1 2"(255) -> ()
          }
          frame 4 {
            n219 = local write "BTR0 2"(9) -> ()
            n220 = local write "BTR1 2"(28) -> ()
          }
          frame 5 {
            n221 = local write "BTR0 2"(131) -> ()
            n222 = local write "BTR1 2"(255) -> ()
          }
          frame 6 {
            n223 = local write "BTR0 2"(4) -> ()
            n224 = local write "BTR1 2"(28) -> ()
          }
          frame 7 {
            n225 = local write "BTR0 2"(3) -> ()
            n226 = local write "BTR1 2"(28) -> ()
          }
          frame 8 {
            n227 = local write "BTR0 2"(129) -> ()
            n228 = local write "BTR1 2"(250) -> ()
          }
          frame 9 {
            n229 = local write "BTR0 2"(1) -> ()
            n230 = local write "BTR1 2"(28) -> ()
          }
          frame 10 {
            n231 = local write "BTR0 2"(128) -> ()
            n232 = local write "BTR1 2"(250) -> ()
          }
          frame 11 {
            n233 = local write "BTR0 2"(0) -> ()
            n234 = local write "BTR1 2"(28) -> ()
          }
          frame 12 {
            n235 = local write "BTR0 2"(128) -> ()
            n236 = local write "BTR1 2"(182) -> ()
          }
          frame 13 {
            n237 = local write "BTR0 2"(0) -> ()
            n238 = local write "BTR1 2"(22) -> ()
          }
          frame 14 {
            n239 = local write "BTR0 2"(0) -> ()
            n240 = local write "BTR1 2"(20) -> ()
          }
          frame 15, Default {
            n241 = local write "BTR0 2"(1) -> ()
            n242 = local write "BTR1 2"(1) -> ()
          }
        }
      }
      event "Radio_Baud": Value Change {
        n243 = event-data() -> ()  [unwired: 7 out]
        n244 = local read "Radio_Baud"() -> (w293:bool)
        n245 = case shown="真" w293 {
          frame False {
            n246 = property on="BTR1" class="DigNum (严格)"("Disabled"=2) -> ()  [unwired: 2 in, 2 out]
            n247 = property on="BTR0" class="DigNum (严格)"("Disabled"=2) -> ()  [unwired: 2 in, 2 out]
            n248 = property on="Baud" class="Ring (严格)"("Disabled"=0) -> ()  [unwired: 2 in, 2 out]
          }
          frame True {
            n249 = property on="BTR0" class="DigNum (严格)"("Disabled"=0) -> ()  [unwired: 2 in, 2 out]
            n250 = property on="BTR1" class="DigNum (严格)"("Disabled"=0) -> ()  [unwired: 2 in, 2 out]
            n251 = property on="Baud" class="Ring (严格)"("Disabled"=2) -> ()  [unwired: 2 in, 2 out]
          }
        }
      }
      event "stop": Value Change {
        n252 = event-data() -> ()  [unwired: 2 out]
        n253 = stacked-sequence {
          tunnel: [_ _ "stop"] -> w300
          frame #0 {
            n254 = local read "DeviceOpen"() -> (w301:bool)
            n255 = case shown="真" w301 {
              frame False {
              }
              frame True {
                w302 = u8 0 ("Disabled")
                n256 = local read "设备类型"() -> (w304:u32)
                n257 = property on="设备类型" class="Ring (严格)"("禁用"=w302) -> ()  [unwired: 2 in, 2 out]
                n258 = dll-call lib="PTH2Kabs J2车用永磁同步电机测试上位机CAN2_源码ControlCAN.dll" fn="VCI_CloseDevice"("DeviceType"=w304, "DeviceInd"=0) -> (w306:u32)  [unwired: 5 in, 2 out]
                n259 = property on="索引" class="Ring (严格)"("Disabled"=w302) -> ()  [unwired: 2 in, 2 out]
                n260 = Equal?(x=w306, y=u32 1) -> (x = y?=w303:bool)
                n261 = case shown="真" w303 {
                  frame False {
                  }
                  frame True {
                    w308 = FALSE ("DeviceOpen")
                    n262 = local write "CANStartup 2"(w308) -> ()
                    n263 = local write "DeviceOpen"(w308) -> ()
                    n264 = local write "CANStartup"(w308) -> ()
                    n265 = property on="OpenDevice" class="Bool"("布尔文本.文本"="打开设备" ("Boolean Text.Text")) -> ()  [unwired: 2 in, 2 out]
                  }
                }
              }
            }
          }
          frame #1 {
            n266 = Wait Until Next ms Multiple(millisecond multiple=u32 500) -> ()  [unwired: 1 out]
            "stop 2" <- TRUE ("stop 2")
          }
          frame #2 {
          }
        }
      }
      event "OpenDevice": Value Change {
        n267 = event-data() -> ()  [unwired: 2 out]
        n268 = case shown="假" "DeviceOpen" {
          frame False {
            w319 = u32 12 items=["PCI5121"=1, "PCI9810"=2, "USBCAN1"=3, "USBCAN2"=4, "PCI9820"=5, "PCI5110"=7, "CANLite(mini)"=8, "ISA9620"=9, "ISA5420"=10, "PC104CAN"=11, "CANETUDP"=12, "DNP9810"=13, "PCI9840B"=14, "PC104C2"=15, "PCI9820I"=16, "CANETTCP"=17, "pec9920"=18, "PCI5010U"=19, "USBCAN_E_U"=20, "USBCAN_2E_U"=21, "PCI5020U"=22] ("DeviceType")
            # "判断使用canet udp模式"
            n269 = local read "设备类型"() -> (w324:u32)
            n270 = local read "设备类型"() -> (w320:u32)
            n271 = local read "本机端口"() -> (w318:u32)
            n272 = Equal?(x=w320, y=w319) -> (x = y?=w314:bool)
            n273 = Select(t=w318, s=w314, f=u32 0) -> (s? t:f=w316:u32)
            n274 = dll-call lib="PTH2Kabs J2车用永磁同步电机测试上位机CAN2_源码ControlCAN.dll" fn="VCI_OpenDevice"("DevType"=w324, "DevIndex"=0, "Reserved"=w316) -> (w323:u32)  [unwired: 6 in, 2 out]
            n275 = Equal?(x=w323, y=u32 1) -> (x = y?=w321:bool)
            n276 = case shown="真" w321 {
              frame False {
                n277 = call "显示对话框信息7"() -> ()  [unwired: 3 in, 9 out]
              }
              frame True {
                n278 = stacked-sequence {
                  seq-local: [w326 _ _ _ _ _ _ _ _] -> [_ w338 _ w371 _ _ _ _ _]
                  frame #0 {
                    w331 = u32 19 items=["PCI5121"=1, "PCI9810"=2, "USBCAN1"=3, "USBCAN2"=4, "PCI9820"=5, "PCI5110"=7, "CANLite(mini)"=8, "ISA9620"=9, "ISA5420"=10, "PC104CAN"=11, "DNP9810"=13, "PCI9840B"=14, "PC104C2"=15, "PCI9820I"=16, "pec9920"=18, "PCI5010U"=19, "USBCAN_E_U"=20, "USBCAN_2E_U"=21, "PCI5020U"=22, ""=0] ("DeviceType")
                    w333 = u32 22 items=["PCI5121"=1, "PCI9810"=2, "USBCAN1"=3, "USBCAN2"=4, "PCI9820"=5, "PCI5110"=7, "CANLite(mini)"=8, "ISA9620"=9, "ISA5420"=10, "PC104CAN"=11, "DNP9810"=13, "PCI9840B"=14, "PC104C2"=15, "PCI9820I"=16, "pec9920"=18, "PCI5010U"=19, "USBCAN_E_U"=20, "USBCAN_2E_U"=21, "PCI5020U"=22, ""=0] ("DeviceType")
                    w325 = TRUE ("ret_ok")
                    w336 = u32 21 items=["PCI5121"=1, "PCI9810"=2, "USBCAN1"=3, "USBCAN2"=4, "PCI9820"=5, "PCI5110"=7, "CANLite(mini)"=8, "ISA9620"=9, "ISA5420"=10, "PC104CAN"=11, "DNP9810"=13, "PCI9840B"=14, "PC104C2"=15, "PCI9820I"=16, "pec9920"=18, "USBCAN_E_U"=20, "USBCAN_2E_U"=21, ""=0] ("DeviceType")
                    w337 = u32 20 items=["PCI5121"=1, "PCI9810"=2, "USBCAN1"=3, "USBCAN2"=4, "PCI9820"=5, "PCI5110"=7, "CANLite(mini)"=8, "ISA9620"=9, "ISA5420"=10, "PC104CAN"=11, "DNP9810"=13, "PCI9840B"=14, "PC104C2"=15, "PCI9820I"=16, "pec9920"=18, "USBCAN_E_U"=20, "USBCAN_2E_U"=21, ""=0] ("DeviceType")
                    # "判断是不是USB_U_E设备"
                    n279 = local read "设备类型"() -> (w332:u32)
                    n280 = Equal?(x=w332, y=w337) -> (x = y?=w335:bool)
                    n281 = Equal?(x=w332, y=w336) -> (x = y?=w334:bool)
                    n282 = Equal?(x=w332, y=w333) -> (x = y?=w330:bool)
                    n283 = Equal?(x=w332, y=w331) -> (x = y?=w329:bool)
                    n284 = Or(x=w335, y=w334) -> (x .or. y?=w328:bool)
                    n285 = Or(x=w330, y=w329) -> (x .or. y?=w327:bool)
                    n286 = Or(x=w328, y=w327) -> (x .or. y?=w326:bool)
                    n287 = local write "retok0"(w325) -> ()
                    n288 = local write "retok1"(w325) -> ()
                  }
                  frame #1 {
                    n289 = case shown="真" w338 {
                      frame False {
                        # "不是 -U-E 设备，不做处理"
                      }
                      frame True {
                        # "USB-E-U初始化"
                        n290 = local read "CAN通道0"() -> (w349:u32)
                        n291 = local read "设备类型"() -> (w347:u32)
                        n292 = local read "索引"() -> (w346:u32)
                        n293 = local read "e-u-baud"() -> (w350:cluster{"数值":u32})
                        n294 = local read "e-u-baud 2"() -> (w343:cluster{"数值":u32})
                        n295 = local read "CAN 通道 2"() -> (w345:u32)
                        n296 = dll-call lib="PTH2Kabs J2车用永磁同步电机测试上位机CAN2_源码ControlCAN.dll" fn="VCI_SetReference"("DevType"=w347, "DevIndex"=w346, "CANInd"=w345, "RefType"=0, "pData"=w343) -> ("返回类型"=w341:u32)  [unwired: 8 in, 2 out]
                        n297 = dll-call lib="PTH2Kabs J2车用永磁同步电机测试上位机CAN2_源码ControlCAN.dll" fn="VCI_SetReference"("DevType"=w347, "DevIndex"=w346, "CANInd"=w349, "RefType"=u32 0 ("y"), "pData"=w350) -> ("返回类型"=w352:u32)  [unwired: 8 in, 2 out]
                        n298 = Equal?(x=w352, y=u32 1) -> (x = y?=w340:bool)
                        n299 = Equal?(x=w341, y=u32 1) -> (x = y?=w339:bool)
                        n300 = local write "retok1"(w339) -> ()
                        n301 = case shown="假" w339 {
                          frame False {
                            n302 = call "显示对话框信息12"() -> ()  [unwired: 3 in, 9 out]
                          }
                          frame True {
                          }
                        }
                        n303 = local write "retok0"(w340) -> ()
                        n304 = case shown="假" w340 {
                          frame False {
                            n305 = call "显示对话框信息3"() -> ()  [unwired: 3 in, 9 out]
                          }
                          frame True {
                          }
                        }
                      }
                    }
                  }
                  frame #2 {
                    n306 = local read "retok1"() -> (w354:bool)
                    n307 = local read "retok0"() -> (w353:bool)
                    n308 = case shown="真" w354 {
                      frame False {
                      }
                      frame True {
                        n309 = local read "CAN 通道 2"() -> (w363:u32)
                        n310 = local read "索引"() -> (w368:u32)
                        n311 = local read "设备类型"() -> (w364:u32)
                        n312 = local read "VCI_INIT_CONFIG"() -> (w365:T1)
                        n313 = dll-call lib="PTH2Kabs J2车用永磁同步电机测试上位机CAN2_源码ControlCAN.dll" fn="VCI_InitCAN"("DeviceType"=w364, "DeviceInd"=w368, "CANInd"=w363, "VCI_INIT_CONFIG"=w365) -> (w366:u32)  [unwired: 7 in, 2 out]
                        n314 = Equal?(x=w366, y=u32 1) -> (x = y?=w362:bool)
                        n315 = local write "retok1"(w362) -> ()
                        n316 = case shown="假" w362 {
                          frame False {
                            n317 = call "显示对话框信息13"() -> ()  [unwired: 3 in, 9 out]
                          }
                          frame True {
                          }
                        }
                      }
                    }
                    n318 = case shown="真" w353 {
                      frame False {
                      }
                      frame True {
                        n319 = local read "CAN通道0"() -> (w361:u32)
                        n320 = local read "索引"() -> (w356:u32)
                        n321 = local read "设备类型"() -> (w360:u32)
                        n322 = local read "VCI_INIT_CONFIG"() -> (w359:T1)
                        n323 = dll-call lib="PTH2Kabs J2车用永磁同步电机测试上位机CAN2_源码ControlCAN.dll" fn="VCI_InitCAN"("DeviceType"=w360, "DeviceInd"=w356, "CANInd"=w361, "VCI_INIT_CONFIG"=w359) -> (w358:u32)  [unwired: 7 in, 2 out]
                        n324 = Equal?(x=w358, y=u32 1) -> (x = y?=w355:bool)
                        n325 = local write "retok0"(w355) -> ()
                        n326 = case shown="假" w355 {
                          frame False {
                            n327 = call "显示对话框信息6"() -> ()  [unwired: 3 in, 9 out]
                          }
                          frame True {
                          }
                        }
                      }
                    }
                  }
                  frame #3 {
                    n328 = local read "retok0"() -> (w373:bool)
                    n329 = local read "retok1"() -> (w370:bool)
                    n330 = And(x=w371, y=w373) -> (x .and. y?=w372:bool)
                    n331 = And(x=w371, y=w370) -> (x .and. y?=w369:bool)
                    n332 = case shown="真" w372 {
                      frame False {
                      }
                      frame True {
                        w392 = u32 2 items=["标准帧滤波", "扩展帧滤波", "禁能滤波"] ("fiter_mode")
                        # "设置波特率正确，就设置滤波"
                        n333 = local read "滤波模式"() -> (w391:u32)
                        n334 = Not Equal?(x=w391, y=w392) -> (x != y?=w390:bool)
                        n335 = case shown="真" w390 {
                          frame False {
                          }
                          frame True {
                            n336 = stacked-sequence {
                              frame #0 {
                                n337 = local read "VCI_FILTER_RECORD"() -> (w394:cluster{"ExtFrame":u32, "Start":u32, "End":u32})
                                n338 = local read "CAN通道0"() -> (w397:u32)
                                n339 = local read "设备类型"() -> (w396:u32)
                                n340 = local read "索引"() -> (w393:u32)
                                n341 = dll-call lib="PTH2Kabs J2车用永磁同步电机测试上位机CAN2_源码ControlCAN.dll" fn="VCI_SetReference"("DevType"=w396, "DevIndex"=w393, "CANInd"=w397, "RefType"=u32 1, "pData"=w394) -> ()  [unwired: 8 in, 3 out]
                              }
                              frame #1 {
                                n342 = local read "CAN通道0"() -> (w405:u32)
                                n343 = local read "索引"() -> (w399:u32)
                                n344 = local read "设备类型"() -> (w404:u32)
                                n345 = dll-call lib="PTH2Kabs J2车用永磁同步电机测试上位机CAN2_源码ControlCAN.dll" fn="VCI_SetReference"("DevType"=w404, "DevIndex"=w399, "CANInd"=w405, "RefType"=u32 2, "pData"=u32 0 ("RefType")) -> ("返回类型"=w401:u32)  [unwired: 7 in, 3 out]
                                n346 = Equal?(x=w401, y=u32 1) -> (x = y?=w398:bool)
                                n347 = local write "retok0"(w398) -> ()
                                n348 = case shown="假" w398 {
                                frame False {
                                n349 = call "显示对话框信息4"() -> ()  [unwired: 3 in, 9 out]
                                }
                                frame True {
                                }
                                }
                              }
                            }
                          }
                        }
                      }
                    }
                    n350 = case shown="真" w369 {
                      frame False {
                      }
                      frame True {
                        w376 = u32 2 items=["标准帧滤波", "扩展帧滤波", "禁能滤波"] ("fiter_mode")
                        # "设置波特率正确，就设置滤波"
                        n351 = local read "滤波模式"() -> (w375:u32)
                        n352 = Not Equal?(x=w375, y=w376) -> (x != y?=w374:bool)
                        n353 = case shown="真" w374 {
                          frame False {
                          }
                          frame True {
                            n354 = stacked-sequence {
                              frame #0 {
                                n355 = local read "CAN 通道 2"() -> (w377:u32)
                                n356 = local read "VCI_FILTER_RECORD"() -> (w379:cluster{"ExtFrame":u32, "Start":u32, "End":u32})
                                n357 = local read "设备类型"() -> (w381:u32)
                                n358 = local read "索引"() -> (w378:u32)
                                n359 = dll-call lib="PTH2Kabs J2车用永磁同步电机测试上位机CAN2_源码ControlCAN.dll" fn="VCI_SetReference"("DevType"=w381, "DevIndex"=w378, "CANInd"=w377, "RefType"=u32 1, "pData"=w379) -> ()  [unwired: 8 in, 3 out]
                              }
                              frame #1 {
                                n360 = local read "CAN 通道 2"() -> (w383:u32)
                                n361 = local read "索引"() -> (w384:u32)
                                n362 = local read "设备类型"() -> (w389:u32)
                                n363 = dll-call lib="PTH2Kabs J2车用永磁同步电机测试上位机CAN2_源码ControlCAN.dll" fn="VCI_SetReference"("DevType"=w389, "DevIndex"=w384, "CANInd"=w383, "RefType"=u32 2, "pData"=u32 0 ("RefType")) -> ("返回类型"=w386:u32)  [unwired: 7 in, 3 out]
                                n364 = Equal?(x=w386, y=u32 1) -> (x = y?=w382:bool)
                                n365 = local write "retok1"(w382) -> ()
                                n366 = case shown="假" w382 {
                                frame False {
                                n367 = call "显示对话框信息14"() -> ()  [unwired: 3 in, 9 out]
                                }
                                frame True {
                                }
                                }
                              }
                            }
                          }
                        }
                      }
                    }
                  }
                  frame #4 {
                    w414 = u32 17 items=["PCI5121"=1, "PCI9810"=2, "USBCAN1"=3, "USBCAN2"=4, "PCI9820"=5, "PCI5110"=7, "CANLite(mini)"=8, "ISA9620"=9, "ISA5420"=10, "PC104CAN"=11, "CANETUDP"=12, "DNP9810"=13, "PCI9840B"=14, "PC104C2"=15, "PCI9820I"=16, "CANETTCP"=17, "pec9920"=18, "PCI5010U"=19, "USBCAN_E_U"=20, "USBCAN_2E_U"=21, "PCI5020U"=22] ("DeviceType")
                    w415 = u32 12 items=["PCI5121"=1, "PCI9810"=2, "USBCAN1"=3, "USBCAN2"=4, "PCI9820"=5, "PCI5110"=7, "CANLite(mini)"=8, "ISA9620"=9, "ISA5420"=10, "PC104CAN"=11, "CANETUDP"=12, "DNP9810"=13, "PCI9840B"=14, "PC104C2"=15, "PCI9820I"=16, "CANETTCP"=17, "pec9920"=18, "PCI5010U"=19, "USBCAN_E_U"=20, "USBCAN_2E_U"=21, "PCI5020U"=22] ("DeviceType")
                    # "如果是UDP模式 或者是 TCP客户端模式"
                    # "客户端模式"
                    # "canet tcp模式"
                    # "判断使用canet udp模式"
                    n368 = local read "本机类型"() -> (w412:enum32{"Radio Selection 1", "Radio Selection 2"})
                    n369 = local read "设备类型"() -> (w413:u32)
                    n370 = Equal?(x=w413, y=w414) -> (x = y?=w409:bool)
                    n371 = Equal?(x=enum32{"Radio Selection 1", "Radio Selection 2"}."Radio Selection 2", y=w412) -> (x = y?=w410:bool)
                    n372 = Equal?(x=w413, y=w415) -> (x = y?=w408:bool)
                    n373 = And(x=w409, y=w410) -> (x .and. y?=w407:bool)
                    n374 = Or(x=w408, y=w407) -> (x .or. y?=w406:bool)
                    n375 = case shown="真" w406 {
                      frame False {
                      }
                      frame True {
                        n376 = stacked-sequence {
                          frame #0 {
                            # "1 端口命令"
                            # "设置 端口"
                            n377 = local read "CANET 端口"() -> (w419:u32)
                            n378 = local read "CAN通道0"() -> (w424:u32)
                            n379 = local read "索引"() -> (w417:u32)
                            n380 = local read "设备类型"() -> (w423:u32)
                            n381 = call "LongToByteArr.vi"("CANET 端口"=w419) -> ("Array"=w418:u8[])
                            n382 = dll-call lib="PTH2Kabs J2车用永磁同步电机测试上位机CAN2_源码ControlCAN.dll" fn="VCI_SetReference"("DevType"=w423, "DevIndex"=w417, "CANInd"=w424, "RefType"=u32 1, "pData"=w418) -> ("返回类型"=w420:u32)  [unwired: 8 in, 2 out]
                            n383 = Equal?(x=w420, y=u32 1) -> (x = y?=w416:bool)
                            n384 = case shown="假" w416 {
                              frame False {
                                n385 = call "显示对话框信息11"() -> ()  [unwired: 3 in, 9 out]
                              }
                              frame True {
                              }
                            }
                            n386 = local write "retok0"(w416) -> ()
                          }
                          frame #1 {
                            # "0 ip命令"
                            # "设置CANET ip"
                            n387 = local read "CANET IP"() -> (w431:string)
                            n388 = local read "CAN通道0"() -> (w436:u32)
                            n389 = local read "索引"() -> (w426:u32)
                            n390 = local read "设备类型"() -> (w435:u32)
                            n391 = String To Byte Array(string=w431) -> (unsigned byte array=w429:u8[])
                            n392 = Array Size(array=w429) -> (size(s)=w430:i32)
                            n393 = Insert Into Array(array=w429, index=w430, new element=u8 0 ("new element/subarray")) -> (w427:u8[])
                            n394 = dll-call lib="PTH2Kabs J2车用永磁同步电机测试上位机CAN2_源码ControlCAN.dll" fn="VCI_SetReference"("DevType"=w435, "DevIndex"=w426, "CANInd"=w436, "RefType"=u32 0, "pData"=w427) -> ("返回类型"=w433:u32)  [unwired: 8 in, 2 out]
                            n395 = Equal?(x=w433, y=u32 1) -> (x = y?=w425:bool)
                            n396 = case shown="假" w425 {
                              frame False {
                                n397 = call "显示对话框信息8"() -> ()  [unwired: 3 in, 9 out]
                              }
                              frame True {
                              }
                            }
                            n398 = local write "retok0"(w425) -> ()
                          }
                          frame #2 {
                            w438 = u8 0 ("element")
                            # "设置 客户端模式"
                            # "0 模式命令"
                            n399 = local read "CAN通道0"() -> (w444:u32)
                            n400 = local read "索引"() -> (w437:u32)
                            n401 = local read "设备类型"() -> (w443:u32)
                            n402 = Build Array(w438, w438, w438, w438) -> (w439:u8[])
                            n403 = dll-call lib="PTH2Kabs J2车用永磁同步电机测试上位机CAN2_源码ControlCAN.dll" fn="VCI_SetReference"("DevType"=w443, "DevIndex"=w437, "CANInd"=w444, "RefType"=u32 4, "pData"=w439) -> ("返回类型"=w442:u32)  [unwired: 7 in, 3 out]
                            n404 = Equal?(x=w442, y=u32 1) -> ()  [unwired: 1 out]
                          }
                        }
                      }
                    }
                  }
                  frame #5 {
                    w453 = u32 17 items=["PCI5121"=1, "PCI9810"=2, "USBCAN1"=3, "USBCAN2"=4, "PCI9820"=5, "PCI5110"=7, "CANLite(mini)"=8, "ISA9620"=9, "ISA5420"=10, "PC104CAN"=11, "CANETUDP"=12, "DNP9810"=13, "PCI9840B"=14, "PC104C2"=15, "PCI9820I"=16, "CANETTCP"=17, "pec9920"=18, "PCI5010U"=19, "USBCAN_E_U"=20, "USBCAN_2E_U"=21, "PCI5020U"=22] ("DeviceType")
                    w454 = u32 12 items=["PCI5121"=1, "PCI9810"=2, "USBCAN1"=3, "USBCAN2"=4, "PCI9820"=5, "PCI5110"=7, "CANLite(mini)"=8, "ISA9620"=9, "ISA5420"=10, "PC104CAN"=11, "CANETUDP"=12, "DNP9810"=13, "PCI9840B"=14, "PC104C2"=15, "PCI9820I"=16, "CANETTCP"=17, "pec9920"=18, "PCI5010U"=19, "USBCAN_E_U"=20, "USBCAN_2E_U"=21, "PCI5020U"=22] ("DeviceType")
                    # "如果是UDP模式 或者是 TCP客户端模式"
                    # "客户端模式"
                    # "canet tcp模式"
                    # "判断使用canet udp模式"
                    n405 = local read "本机类型"() -> (w451:enum32{"Radio Selection 1", "Radio Selection 2"})
                    n406 = local read "设备类型"() -> (w452:u32)
                    n407 = Equal?(x=w452, y=w453) -> (x = y?=w448:bool)
                    n408 = Equal?(x=enum32{"Radio Selection 1", "Radio Selection 2"}."Radio Selection 2", y=w451) -> (x = y?=w449:bool)
                    n409 = Equal?(x=w452, y=w454) -> (x = y?=w447:bool)
                    n410 = And(x=w448, y=w449) -> (x .and. y?=w446:bool)
                    n411 = Or(x=w447, y=w446) -> (x .or. y?=w445:bool)
                    n412 = case shown="真" w445 {
                      frame False {
                      }
                      frame True {
                        n413 = stacked-sequence {
                          frame #0 {
                            # "1 端口命令"
                            # "设置 端口"
                            n414 = local read "CANET 端口"() -> (w460:u32)
                            n415 = local read "CAN 通道 2"() -> (w456:u32)
                            n416 = local read "索引"() -> (w458:u32)
                            n417 = local read "设备类型"() -> (w463:u32)
                            n418 = call "LongToByteArr.vi"("CANET 端口"=w460) -> ("Array"=w459:u8[])
                            n419 = dll-call lib="PTH2Kabs J2车用永磁同步电机测试上位机CAN2_源码ControlCAN.dll" fn="VCI_SetReference"("DevType"=w463, "DevIndex"=w458, "CANInd"=w456, "RefType"=u32 1, "pData"=w459) -> ("返回类型"=w461:u32)  [unwired: 8 in, 2 out]
                            n420 = Equal?(x=w461, y=u32 1) -> (x = y?=w455:bool)
                            n421 = case shown="假" w455 {
                              frame False {
                                n422 = call "显示对话框信息15"() -> ()  [unwired: 3 in, 9 out]
                              }
                              frame True {
                              }
                            }
                            n423 = local write "retok1"(w455) -> ()
                          }
                          frame #1 {
                            # "0 ip命令"
                            # "设置CANET ip"
                            n424 = local read "CANET IP"() -> (w471:string)
                            n425 = local read "索引"() -> (w466:u32)
                            n426 = local read "设备类型"() -> (w475:u32)
                            n427 = local read "CAN 通道 2"() -> (w464:u32)
                            n428 = String To Byte Array(string=w471) -> (unsigned byte array=w469:u8[])
                            n429 = Array Size(array=w469) -> (size(s)=w470:i32)
                            n430 = Insert Into Array(array=w469, index=w470, new element=u8 0 ("new element/subarray")) -> (w467:u8[])
                            n431 = dll-call lib="PTH2Kabs J2车用永磁同步电机测试上位机CAN2_源码ControlCAN.dll" fn="VCI_SetReference"("DevType"=w475, "DevIndex"=w466, "CANInd"=w464, "RefType"=u32 0, "pData"=w467) -> ("返回类型"=w473:u32)  [unwired: 8 in, 2 out]
                            n432 = Equal?(x=w473, y=u32 1) -> (x = y?=w465:bool)
                            n433 = case shown="假" w465 {
                              frame False {
                                n434 = call "显示对话框信息16"() -> ()  [unwired: 3 in, 9 out]
                              }
                              frame True {
                              }
                            }
                            n435 = local write "retok1"(w465) -> ()
                          }
                          frame #2 {
                            w478 = u8 0 ("element")
                            # "设置 客户端模式"
                            # "0 模式命令"
                            n436 = local read "CAN 通道 2"() -> (w476:u32)
                            n437 = local read "索引"() -> (w477:u32)
                            n438 = local read "设备类型"() -> (w483:u32)
                            n439 = Build Array(w478, w478, w478, w478) -> (w479:u8[])
                            n440 = dll-call lib="PTH2Kabs J2车用永磁同步电机测试上位机CAN2_源码ControlCAN.dll" fn="VCI_SetReference"("DevType"=w483, "DevIndex"=w477, "CANInd"=w476, "RefType"=u32 4, "pData"=w479) -> ("返回类型"=w482:u32)  [unwired: 7 in, 3 out]
                            n441 = Equal?(x=w482, y=u32 1) -> ()  [unwired: 1 out]
                          }
                        }
                      }
                    }
                  }
                  frame #6 {
                    w490 = u32 17 items=["PCI5121"=1, "PCI9810"=2, "USBCAN1"=3, "USBCAN2"=4, "PCI9820"=5, "PCI5110"=7, "CANLite(mini)"=8, "ISA9620"=9, "ISA5420"=10, "PC104CAN"=11, "CANETUDP"=12, "DNP9810"=13, "PCI9840B"=14, "PC104C2"=15, "PCI9820I"=16, "CANETTCP"=17, "pec9920"=18, "PCI5010U"=19, "USBCAN_E_U"=20, "USBCAN_2E_U"=21, "PCI5020U"=22] ("DeviceType")
                    # "服务器模式"
                    # "canet tcp模式"
                    n442 = local read "设备类型"() -> (w485:u32)
                    n443 = local read "本机类型"() -> (w489:enum32{"Radio Selection 1", "Radio Selection 2"})
                    n444 = Equal?(x=w485, y=w490) -> (x = y?=w486:bool)
                    n445 = Equal?(x=enum32{"Radio Selection 1", "Radio Selection 2"}."Radio Selection 1", y=w489) -> (x = y?=w487:bool)
                    n446 = And(x=w486, y=w487) -> (x .and. y?=w484:bool)
                    n447 = case shown="真" w484 {
                      frame False {
                      }
                      frame True {
                        # "如果是 tcp 服务器模式"
                        n448 = stacked-sequence {
                          frame #0 {
                            # "2 本机端口命令"
                            # "设置 服务器 本机端口"
                            n449 = local read "本机端口"() -> (w494:u32)
                            n450 = local read "CAN通道0"() -> (w499:u32)
                            n451 = local read "设备类型"() -> (w498:u32)
                            n452 = local read "索引"() -> (w492:u32)
                            n453 = call "LongToByteArr.vi"("CANET 端口"=w494) -> ("Array"=w493:u8[])
                            n454 = dll-call lib="PTH2Kabs J2车用永磁同步电机测试上位机CAN2_源码ControlCAN.dll" fn="VCI_SetReference"("DevType"=w498, "DevIndex"=w492, "CANInd"=w499, "RefType"=u32 2, "pData"=w493) -> ("返回类型"=w495:u32)  [unwired: 8 in, 2 out]
                            n455 = Equal?(x=w495, y=u32 1) -> (x = y?=w491:bool)
                            n456 = case shown="假" w491 {
                              frame False {
                                n457 = call "显示对话框信息10"() -> ()  [unwired: 3 in, 9 out]
                              }
                              frame True {
                              }
                            }
                            n458 = local write "retok0"(w491) -> ()
                          }
                          frame #1 {
                            # "0 模式命令"
                            # "设置 服务器模式"
                            n459 = local read "CAN通道0"() -> (w507:u32)
                            n460 = local read "设备类型"() -> (w506:u32)
                            n461 = local read "索引"() -> (w501:u32)
                            n462 = local read "type"() -> (w502:u8[])
                            n463 = dll-call lib="PTH2Kabs J2车用永磁同步电机测试上位机CAN2_源码ControlCAN.dll" fn="VCI_SetReference"("DevType"=w506, "DevIndex"=w501, "CANInd"=w507, "RefType"=u32 4, "pData"=w502) -> ("返回类型"=w504:u32)  [unwired: 8 in, 2 out]
                            n464 = Equal?(x=w504, y=u32 1) -> (x = y?=w500:bool)
                            n465 = case shown="假" w500 {
                              frame False {
                                n466 = call "显示对话框信息9"() -> ()  [unwired: 3 in, 9 out]
                              }
                              frame True {
                              }
                            }
                            n467 = local write "retok0"(w500) -> ()
                          }
                        }
                      }
                    }
                  }
                  frame #7 {
                    w514 = u32 17 items=["PCI5121"=1, "PCI9810"=2, "USBCAN1"=3, "USBCAN2"=4, "PCI9820"=5, "PCI5110"=7, "CANLite(mini)"=8, "ISA9620"=9, "ISA5420"=10, "PC104CAN"=11, "CANETUDP"=12, "DNP9810"=13, "PCI9840B"=14, "PC104C2"=15, "PCI9820I"=16, "CANETTCP"=17, "pec9920"=18, "PCI5010U"=19, "USBCAN_E_U"=20, "USBCAN_2E_U"=21, "PCI5020U"=22] ("DeviceType")
                    # "服务器模式"
                    # "canet tcp模式"
                    n468 = local read "设备类型"() -> (w509:u32)
                    n469 = local read "本机类型"() -> (w513:enum32{"Radio Selection 1", "Radio Selection 2"})
                    n470 = Equal?(x=w509, y=w514) -> (x = y?=w510:bool)
                    n471 = Equal?(x=enum32{"Radio Selection 1", "Radio Selection 2"}."Radio Selection 1", y=w513) -> (x = y?=w511:bool)
                    n472 = And(x=w510, y=w511) -> (x .and. y?=w508:bool)
                    n473 = case shown="真" w508 {
                      frame False {
                      }
                      frame True {
                        # "如果是 tcp 服务器模式"
                        n474 = stacked-sequence {
                          frame #0 {
                            # "2 本机端口命令"
                            # "设置 服务器 本机端口"
                            n475 = local read "CAN 通道 2"() -> (w515:u32)
                            n476 = local read "本机端口"() -> (w519:u32)
                            n477 = local read "设备类型"() -> (w523:u32)
                            n478 = local read "索引"() -> (w517:u32)
                            n479 = call "LongToByteArr.vi"("CANET 端口"=w519) -> ("Array"=w518:u8[])
                            n480 = dll-call lib="PTH2Kabs J2车用永磁同步电机测试上位机CAN2_源码ControlCAN.dll" fn="VCI_SetReference"("DevType"=w523, "DevIndex"=w517, "CANInd"=w515, "RefType"=u32 2, "pData"=w518) -> ("返回类型"=w520:u32)  [unwired: 8 in, 2 out]
                            n481 = Equal?(x=w520, y=u32 1) -> (x = y?=w516:bool)
                            n482 = case shown="假" w516 {
                              frame False {
                                n483 = call "显示对话框信息17"() -> ()  [unwired: 3 in, 9 out]
                              }
                              frame True {
                              }
                            }
                            n484 = local write "retok1"(w516) -> ()
                          }
                          frame #1 {
                            # "0 模式命令"
                            # "设置 服务器模式"
                            n485 = local read "CAN 通道 2"() -> (w524:u32)
                            n486 = local read "设备类型"() -> (w531:u32)
                            n487 = local read "索引"() -> (w526:u32)
                            n488 = local read "type"() -> (w527:u8[])
                            n489 = dll-call lib="PTH2Kabs J2车用永磁同步电机测试上位机CAN2_源码ControlCAN.dll" fn="VCI_SetReference"("DevType"=w531, "DevIndex"=w526, "CANInd"=w524, "RefType"=u32 4, "pData"=w527) -> ("返回类型"=w529:u32)  [unwired: 8 in, 2 out]
                            n490 = Equal?(x=w529, y=u32 1) -> (x = y?=w525:bool)
                            n491 = case shown="假" w525 {
                              frame False {
                                n492 = call "显示对话框信息18"() -> ()  [unwired: 3 in, 9 out]
                              }
                              frame True {
                              }
                            }
                            n493 = local write "retok1"(w525) -> ()
                          }
                        }
                      }
                    }
                  }
                  frame #8 {
                    n494 = local read "retok0"() -> (w534:bool)
                    n495 = local read "retok1"() -> (w533:bool)
                    n496 = And(x=w534, y=w533) -> (x .and. y?=w532:bool)
                    n497 = case shown="真" w532 {
                      frame False {
                        n498 = local read "设备类型"() -> (w536:u32)
                        n499 = local read "索引"() -> (w535:u32)
                        n500 = dll-call lib="PTH2Kabs J2车用永磁同步电机测试上位机CAN2_源码ControlCAN.dll" fn="VCI_CloseDevice"("DeviceType"=w536, "DeviceInd"=w535) -> ()  [unwired: 5 in, 3 out]
                        n501 = call "显示对话框信息5"() -> ()  [unwired: 3 in, 9 out]
                      }
                      frame True {
                        n502 = property on="OpenDevice" class="Bool"("布尔文本.文本"="关闭设备") -> ()  [unwired: 2 in, 2 out]
                        n503 = property on="设备类型" class="Ring (严格)"("禁用"=u8 0 ("Disabled")) -> ()  [unwired: 2 in, 2 out]
                        n504 = call <vilib>:"Application Directory.vi"() -> ("Application Directory"=w539:path)
                        n505 = local write "DeviceOpen"(TRUE ("DeviceOpen")) -> ()
                        n506 = Strip Path(path=w539) -> (stripped path=w540:path)  [unwired: 1 out]
                        n507 = Format Date/Time String(time format string (%c)="%Y%m%d%H%M%S", UTC format=FALSE) -> (date/time string=w543:string)  [unwired: 1 in]
                        n508 = Concatenate Strings("Test", w543, ".csv") -> (w538:string)
                        n509 = Build Path(base path=w540, name or relative path=w538) -> (appended path=w537:path)
                        n510 = local write "保存路径 2"(w537) -> ()
                      }
                    }
                  }
                }
              }
            }
          }
          frame True {
            n511 = stacked-sequence {
              frame #0 {
                n512 = local read "设备类型"() -> (w552:u32)
                n513 = dll-call lib="PTH2Kabs J2车用永磁同步电机测试上位机CAN2_源码ControlCAN.dll" fn="VCI_CloseDevice"("DeviceType"=w552, "DeviceInd"=0) -> (w551:u32)  [unwired: 5 in, 2 out]
                n514 = Equal?(x=w551, y=u32 1) -> (x = y?=w549:bool)
                n515 = case shown="真" w549 {
                  frame False {
                  }
                  frame True {
                    w555 = u8 0 ("Disabled")
                    w554 = FALSE
                    n516 = property on="OpenDevice" class="Bool"("布尔文本.文本"="打开设备" ("Boolean Text.Text")) -> ()  [unwired: 2 in, 2 out]
                    n517 = local write "CANStartup 2"(w554) -> ()
                    n518 = local write "CANStartup"(w554) -> ()
                    n519 = local write "DeviceOpen"(w554) -> ()
                    n520 = property on="设备类型" class="Ring (严格)"("禁用"=w555) -> ()  [unwired: 2 in, 2 out]
                    n521 = property on="索引" class="Ring (严格)"("Disabled"=w555) -> ()  [unwired: 2 in, 2 out]
                  }
                }
              }
              frame #1 {
                w565 = u32 19 items=["PCI5121"=1, "PCI9810"=2, "USBCAN1"=3, "USBCAN2"=4, "PCI9820"=5, "PCI5110"=7, "CANLite(mini)"=8, "ISA9620"=9, "ISA5420"=10, "PC104CAN"=11, "DNP9810"=13, "PCI9840B"=14, "PC104C2"=15, "PCI9820I"=16, "pec9920"=18, "PCI5010U"=19, "USBCAN_E_U"=20, "USBCAN_2E_U"=21, "PCI5020U"=22, ""=0] ("DeviceType")
                w566 = u32 22 items=["PCI5121"=1, "PCI9810"=2, "USBCAN1"=3, "USBCAN2"=4, "PCI9820"=5, "PCI5110"=7, "CANLite(mini)"=8, "ISA9620"=9, "ISA5420"=10, "PC104CAN"=11, "DNP9810"=13, "PCI9840B"=14, "PC104C2"=15, "PCI9820I"=16, "pec9920"=18, "PCI5010U"=19, "USBCAN_E_U"=20, "USBCAN_2E_U"=21, "PCI5020U"=22, ""=0] ("DeviceType")
                w567 = u32 21 items=["PCI5121"=1, "PCI9810"=2, "USBCAN1"=3, "USBCAN2"=4, "PCI9820"=5, "PCI5110"=7, "CANLite(mini)"=8, "ISA9620"=9, "ISA5420"=10, "PC104CAN"=11, "DNP9810"=13, "PCI9840B"=14, "PC104C2"=15, "PCI9820I"=16, "pec9920"=18, "USBCAN_E_U"=20, "USBCAN_2E_U"=21, ""=0] ("DeviceType")
                w568 = u32 20 items=["PCI5121"=1, "PCI9810"=2, "USBCAN1"=3, "USBCAN2"=4, "PCI9820"=5, "PCI5110"=7, "CANLite(mini)"=8, "ISA9620"=9, "ISA5420"=10, "PC104CAN"=11, "DNP9810"=13, "PCI9840B"=14, "PC104C2"=15, "PCI9820I"=16, "pec9920"=18, "USBCAN_E_U"=20, "USBCAN_2E_U"=21, ""=0] ("DeviceType")
                n522 = local read "设备类型"() -> (w564:u32)
                n523 = Equal?(x=w564, y=w568) -> (x = y?=w563:bool)
                n524 = Equal?(x=w564, y=w567) -> (x = y?=w562:bool)
                n525 = Equal?(x=w564, y=w566) -> (x = y?=w561:bool)
                n526 = Equal?(x=w564, y=w565) -> (x = y?=w560:bool)
                n527 = Or(x=w561, y=w560) -> (x .or. y?=w558:bool)
                n528 = Or(x=w563, y=w562) -> (x .or. y?=w559:bool)
                n529 = Or(x=w559, y=w558) -> (x .or. y?=w557:bool)
                n530 = case shown="假" w557 {
                  frame False {
                    n531 = local read "Baud 2"() -> (w569:u32)
                    n532 = local read "Baud"() -> (w570:u32)
                    n533 = case shown="0" w569 {
                      frame 0 {
                        n534 = local write "BTR0 2"(u8 191 ("BTR0")) -> ()
                        n535 = local write "BTR1 2"(u8 255 ("BTR1")) -> ()
                      }
                      frame 1 {
                        n536 = local write "BTR0 2"(49) -> ()
                        n537 = local write "BTR1 2"(28) -> ()
                      }
                      frame 2 {
                        n538 = local write "BTR0 2"(24) -> ()
                        n539 = local write "BTR1 2"(28) -> ()
                      }
                      frame 3 {
                        n540 = local write "BTR0 2"(135) -> ()
                        n541 = local write "BTR1 2"(255) -> ()
                      }
                      frame 4 {
                        n542 = local write "BTR0 2"(9) -> ()
                        n543 = local write "BTR1 2"(28) -> ()
                      }
                      frame 5 {
                        n544 = local write "BTR0 2"(131) -> ()
                        n545 = local write "BTR1 2"(255) -> ()
                      }
                      frame 6 {
                        n546 = local write "BTR0 2"(4) -> ()
                        n547 = local write "BTR1 2"(28) -> ()
                      }
                      frame 7 {
                        n548 = local write "BTR0 2"(3) -> ()
                        n549 = local write "BTR1 2"(28) -> ()
                      }
                      frame 8 {
                        n550 = local write "BTR0 2"(129) -> ()
                        n551 = local write "BTR1 2"(250) -> ()
                      }
                      frame 9 {
                        n552 = local write "BTR0 2"(1) -> ()
                        n553 = local write "BTR1 2"(28) -> ()
                      }
                      frame 10 {
                        n554 = local write "BTR0 2"(128) -> ()
                        n555 = local write "BTR1 2"(250) -> ()
                      }
                      frame 11 {
                        n556 = local write "BTR0 2"(0) -> ()
                        n557 = local write "BTR1 2"(28) -> ()
                      }
                      frame 12 {
                        n558 = local write "BTR0 2"(128) -> ()
                        n559 = local write "BTR1 2"(182) -> ()
                      }
                      frame 13 {
                        n560 = local write "BTR0 2"(0) -> ()
                        n561 = local write "BTR1 2"(22) -> ()
                      }
                      frame 14 {
                        n562 = local write "BTR0 2"(0) -> ()
                        n563 = local write "BTR1 2"(20) -> ()
                      }
                      frame 15, Default {
                        n564 = local write "BTR0 2"(1) -> ()
                        n565 = local write "BTR1 2"(1) -> ()
                      }
                    }
                    n566 = case shown="0" w570 {
                      frame 0 {
                        n567 = local write "BTR0"(u8 191 ("BTR0")) -> ()
                        n568 = local write "BTR1"(u8 255 ("BTR1")) -> ()
                      }
                      frame 1 {
                        n569 = local write "BTR0"(u8 49 ("BTR0")) -> ()
                        n570 = local write "BTR1"(u8 28 ("BTR1")) -> ()
                      }
                      frame 2 {
                        n571 = local write "BTR0"(u8 24 ("BTR0")) -> ()
                        n572 = local write "BTR1"(u8 28 ("BTR1")) -> ()
                      }
                      frame 3 {
                        n573 = local write "BTR1"(u8 255 ("BTR1")) -> ()
                        n574 = local write "BTR0"(u8 135 ("BTR0")) -> ()
                      }
                      frame 4 {
                        n575 = local write "BTR1"(u8 28 ("BTR1")) -> ()
                        n576 = local write "BTR0"(u8 9 ("BTR0")) -> ()
                      }
                      frame 5 {
                        n577 = local write "BTR0"(u8 131 ("BTR0")) -> ()
                        n578 = local write "BTR1"(u8 255 ("BTR1")) -> ()
                      }
                      frame 6 {
                        n579 = local write "BTR1"(u8 28 ("BTR1")) -> ()
                        n580 = local write "BTR0"(u8 4 ("BTR0")) -> ()
                      }
                      frame 7 {
                        n581 = local write "BTR0"(u8 3 ("BTR0")) -> ()
                        n582 = local write "BTR1"(u8 28 ("BTR1")) -> ()
                      }
                      frame 8 {
                        n583 = local write "BTR0"(u8 129 ("BTR0")) -> ()
                        n584 = local write "BTR1"(u8 250 ("BTR1")) -> ()
                      }
                      frame 9 {
                        n585 = local write "BTR1"(u8 28 ("BTR1")) -> ()
                        n586 = local write "BTR0"(u8 1 ("BTR0")) -> ()
                      }
                      frame 10 {
                        n587 = local write "BTR0"(u8 128 ("BTR0")) -> ()
                        n588 = local write "BTR1"(u8 250 ("BTR1")) -> ()
                      }
                      frame 11 {
                        n589 = local write "BTR0"(u8 0 ("BTR0")) -> ()
                        n590 = local write "BTR1"(u8 28 ("BTR1")) -> ()
                      }
                      frame 12 {
                        n591 = local write "BTR0"(u8 128 ("BTR0")) -> ()
                        n592 = local write "BTR1"(u8 182 ("BTR1")) -> ()
                      }
                      frame 13 {
                        n593 = local write "BTR1"(u8 22 ("BTR1")) -> ()
                        n594 = local write "BTR0"(u8 0 ("BTR0")) -> ()
                      }
                      frame 14 {
                        n595 = local write "BTR0"(u8 0 ("BTR0")) -> ()
                        n596 = local write "BTR1"(u8 20 ("BTR1")) -> ()
                      }
                      frame 15, Default {
                      }
                    }
                  }
                  frame True {
                    w633 = 0
                    n597 = local write "Radio_Baud(E_U)"(FALSE) -> ()
                    n598 = local write "BTR0 2"(w633) -> ()
                    n599 = local write "BTR1 2"(w633) -> ()
                    n600 = local write "BTR1"(w633) -> ()
                    n601 = local write "BTR0"(w633) -> ()
                  }
                }
              }
            }
          }
        }
      }
      event "设备类型": Value Change {
        w641 = u32 22 items=["PCI5121"=1, "PCI9810"=2, "USBCAN1"=3, "USBCAN2"=4, "PCI9820"=5, "PCI5110"=7, "CANLite(mini)"=8, "ISA9620"=9, "ISA5420"=10, "PC104CAN"=11, "DNP9810"=13, "PCI9840B"=14, "PC104C2"=15, "PCI9820I"=16, "pec9920"=18, "PCI5010U"=19, "USBCAN_E_U"=20, "USBCAN_2E_U"=21, "PCI5020U"=22, ""=0] ("DeviceType")
        w642 = u32 19 items=["PCI5121"=1, "PCI9810"=2, "USBCAN1"=3, "USBCAN2"=4, "PCI9820"=5, "PCI5110"=7, "CANLite(mini)"=8, "ISA9620"=9, "ISA5420"=10, "PC104CAN"=11, "DNP9810"=13, "PCI9840B"=14, "PC104C2"=15, "PCI9820I"=16, "pec9920"=18, "PCI5010U"=19, "USBCAN_E_U"=20, "USBCAN_2E_U"=21, "PCI5020U"=22, ""=0] ("DeviceType")
        w645 = u32 21 items=["PCI5121"=1, "PCI9810"=2, "USBCAN1"=3, "USBCAN2"=4, "PCI9820"=5, "PCI5110"=7, "CANLite(mini)"=8, "ISA9620"=9, "ISA5420"=10, "PC104CAN"=11, "DNP9810"=13, "PCI9840B"=14, "PC104C2"=15, "PCI9820I"=16, "pec9920"=18, "USBCAN_E_U"=20, "USBCAN_2E_U"=21, ""=0] ("DeviceType")
        w646 = u32 20 items=["PCI5121"=1, "PCI9810"=2, "USBCAN1"=3, "USBCAN2"=4, "PCI9820"=5, "PCI5110"=7, "CANLite(mini)"=8, "ISA9620"=9, "ISA5420"=10, "PC104CAN"=11, "DNP9810"=13, "PCI9840B"=14, "PC104C2"=15, "PCI9820I"=16, "pec9920"=18, "USBCAN_E_U"=20, "USBCAN_2E_U"=21, ""=0] ("DeviceType")
        n602 = event-data() -> ()  [unwired: 7 out]
        n603 = local read "设备类型"() -> (w640:u32)
        n604 = Equal?(x=w641, y=w640) -> (x = y?=w638:bool)
        n605 = Equal?(x=w640, y=w646) -> (x = y?=w644:bool)
        n606 = Equal?(x=w640, y=w645) -> (x = y?=w643:bool)
        n607 = Equal?(x=w642, y=w640) -> (x = y?=w639:bool)
        n608 = Or(x=w639, y=w638) -> (x .or. y?=w636:bool)
        n609 = Or(x=w644, y=w643) -> (x .or. y?=w637:bool)
        n610 = Or(x=w637, y=w636) -> (x .or. y?=w635:bool)
        n611 = case shown="假" w635 {
          frame False {
            n612 = stacked-sequence {
              frame #0 {
                n613 = local write "Radio_Baud"(FALSE) -> ()
              }
              frame #1 {
                n614 = local read "Baud"() -> (w649:u32)
                n615 = case shown="0" w649 {
                  frame 0 {
                    n616 = local write "BTR0"(u8 191 ("BTR0")) -> ()
                    n617 = local write "BTR1"(u8 255 ("BTR1")) -> ()
                  }
                  frame 1 {
                    n618 = local write "BTR0"(u8 49 ("BTR0")) -> ()
                    n619 = local write "BTR1"(u8 28 ("BTR1")) -> ()
                  }
                  frame 2 {
                    n620 = local write "BTR0"(u8 24 ("BTR0")) -> ()
                    n621 = local write "BTR1"(u8 28 ("BTR1")) -> ()
                  }
                  frame 3 {
                    n622 = local write "BTR1"(u8 255 ("BTR1")) -> ()
                    n623 = local write "BTR0"(u8 135 ("BTR0")) -> ()
                  }
                  frame 4 {
                    n624 = local write "BTR1"(u8 28 ("BTR1")) -> ()
                    n625 = local write "BTR0"(u8 9 ("BTR0")) -> ()
                  }
                  frame 5 {
                    n626 = local write "BTR0"(u8 131 ("BTR0")) -> ()
                    n627 = local write "BTR1"(u8 255 ("BTR1")) -> ()
                  }
                  frame 6 {
                    n628 = local write "BTR1"(u8 28 ("BTR1")) -> ()
                    n629 = local write "BTR0"(u8 4 ("BTR0")) -> ()
                  }
                  frame 7 {
                    n630 = local write "BTR0"(u8 3 ("BTR0")) -> ()
                    n631 = local write "BTR1"(u8 28 ("BTR1")) -> ()
                  }
                  frame 8 {
                    n632 = local write "BTR0"(u8 129 ("BTR0")) -> ()
                    n633 = local write "BTR1"(u8 250 ("BTR1")) -> ()
                  }
                  frame 9 {
                    n634 = local write "BTR1"(u8 28 ("BTR1")) -> ()
                    n635 = local write "BTR0"(u8 1 ("BTR0")) -> ()
                  }
                  frame 10 {
                    n636 = local write "BTR0"(u8 128 ("BTR0")) -> ()
                    n637 = local write "BTR1"(u8 250 ("BTR1")) -> ()
                  }
                  frame 11 {
                    n638 = local write "BTR0"(u8 0 ("BTR0")) -> ()
                    n639 = local write "BTR1"(u8 28 ("BTR1")) -> ()
                  }
                  frame 12 {
                    n640 = local write "BTR0"(u8 128 ("BTR0")) -> ()
                    n641 = local write "BTR1"(u8 182 ("BTR1")) -> ()
                  }
                  frame 13 {
                    n642 = local write "BTR1"(u8 22 ("BTR1")) -> ()
                    n643 = local write "BTR0"(u8 0 ("BTR0")) -> ()
                  }
                  frame 14 {
                    n644 = local write "BTR0"(u8 0 ("BTR0")) -> ()
                    n645 = local write "BTR1"(u8 20 ("BTR1")) -> ()
                  }
                  frame 15, Default {
                  }
                }
                n646 = local read "Baud 2"() -> (w648:u32)
                n647 = case shown="0" w648 {
                  frame 0 {
                    n648 = local write "BTR0 2"(u8 191 ("BTR0")) -> ()
                    n649 = local write "BTR1 2"(u8 255 ("BTR1")) -> ()
                  }
                  frame 1 {
                    n650 = local write "BTR0 2"(49) -> ()
                    n651 = local write "BTR1 2"(28) -> ()
                  }
                  frame 2 {
                    n652 = local write "BTR0 2"(24) -> ()
                    n653 = local write "BTR1 2"(28) -> ()
                  }
                  frame 3 {
                    n654 = local write "BTR0 2"(135) -> ()
                    n655 = local write "BTR1 2"(255) -> ()
                  }
                  frame 4 {
                    n656 = local write "BTR0 2"(9) -> ()
                    n657 = local write "BTR1 2"(28) -> ()
                  }
                  frame 5 {
                    n658 = local write "BTR0 2"(131) -> ()
                    n659 = local write "BTR1 2"(255) -> ()
                  }
                  frame 6 {
                    n660 = local write "BTR0 2"(4) -> ()
                    n661 = local write "BTR1 2"(28) -> ()
                  }
                  frame 7 {
                    n662 = local write "BTR0 2"(3) -> ()
                    n663 = local write "BTR1 2"(28) -> ()
                  }
                  frame 8 {
                    n664 = local write "BTR0 2"(129) -> ()
                    n665 = local write "BTR1 2"(250) -> ()
                  }
                  frame 9 {
                    n666 = local write "BTR0 2"(1) -> ()
                    n667 = local write "BTR1 2"(28) -> ()
                  }
                  frame 10 {
                    n668 = local write "BTR0 2"(128) -> ()
                    n669 = local write "BTR1 2"(250) -> ()
                  }
                  frame 11 {
                    n670 = local write "BTR0 2"(0) -> ()
                    n671 = local write "BTR1 2"(28) -> ()
                  }
                  frame 12 {
                    n672 = local write "BTR0 2"(128) -> ()
                    n673 = local write "BTR1 2"(182) -> ()
                  }
                  frame 13 {
                    n674 = local write "BTR0 2"(0) -> ()
                    n675 = local write "BTR1 2"(22) -> ()
                  }
                  frame 14 {
                    n676 = local write "BTR0 2"(0) -> ()
                    n677 = local write "BTR1 2"(20) -> ()
                  }
                  frame 15, Default {
                    n678 = local write "BTR0 2"(1) -> ()
                    n679 = local write "BTR1 2"(1) -> ()
                  }
                }
              }
            }
          }
          frame True {
            n680 = stacked-sequence {
              frame #0 {
                w712 = 0
                n681 = local write "BTR0 2"(w712) -> ()
                n682 = local write "BTR1"(w712) -> ()
                n683 = local write "BTR1 2"(w712) -> ()
                n684 = local write "BTR0"(w712) -> ()
                n685 = local write "Radio_Baud(E_U)"(FALSE) -> ()
              }
              frame #1 {
                n686 = local read "Baud 2"() -> (w714:u32)
                n687 = local read "Baud"() -> (w715:u32)
                n688 = case shown="13" w714 {
                  frame 15, Default {
                  }
                  frame 14 {
                    n689 = local write "寄存器 2"(393219) -> ()
                  }
                  frame 13 {
                    n690 = local write "寄存器 2"(393220) -> ()
                  }
                  frame 11 {
                    n691 = local write "寄存器 2"(393223) -> ()
                  }
                  frame 9 {
                    n692 = local write "寄存器 2"(1835016) -> ()
                  }
                  frame 7 {
                    n693 = local write "寄存器 2"(1835025) -> ()
                  }
                  frame 6 {
                    n694 = local write "寄存器 2"(1441827) -> ()
                  }
                  frame 4 {
                    n695 = local write "寄存器 2"(1835052) -> ()
                  }
                  frame 2 {
                    n696 = local write "寄存器 2"(1441971) -> ()
                  }
                  frame 1 {
                    n697 = local write "寄存器 2"(1835232) -> ()
                  }
                  frame 0 {
                    n698 = local write "寄存器 2"(1835457) -> ()
                  }
                }
                n699 = case shown="14" w715 {
                  frame 15, Default {
                  }
                  frame 14 {
                    n700 = local write "寄存器"(393219) -> ()
                  }
                  frame 13 {
                    n701 = local write "寄存器"(393220) -> ()
                  }
                  frame 11 {
                    n702 = local write "寄存器"(393223) -> ()
                  }
                  frame 9 {
                    n703 = local write "寄存器"(1835016) -> ()
                  }
                  frame 7 {
                    n704 = local write "寄存器"(1835025) -> ()
                  }
                  frame 6 {
                    n705 = local write "寄存器"(1441827) -> ()
                  }
                  frame 4 {
                    n706 = local write "寄存器"(1835052) -> ()
                  }
                  frame 2 {
                    n707 = local write "寄存器"(1441971) -> ()
                  }
                  frame 1 {
                    n708 = local write "寄存器"(1835232) -> ()
                  }
                  frame 0 {
                    n709 = local write "寄存器"(1835457) -> ()
                  }
                }
              }
            }
          }
        }
      }
      event "StartCAN": Value Change {
        n710 = event-data() -> ()  [unwired: 7 out]
        n711 = local read "CAN通道0"() -> (w740:u32)
        n712 = local read "设备类型"() -> (w741:u32)
        n713 = local read "索引"() -> (w736:u32)
        n714 = dll-call lib="PTH2Kabs J2车用永磁同步电机测试上位机CAN2_源码ControlCAN.dll" fn="VCI_StartCAN"("DeviceType"=w741, "DeviceInd"=w736, "CANInd"=w740) -> (w739:u32)  [unwired: 6 in, 2 out]
        n715 = Equal?(x=w739, y=u32 1) -> (x = y?=w737:bool)
        n716 = case shown="真" w737 {
          selector: w737 -> [_ w743]
          frame False {
          }
          frame True {
            n717 = property on="索引" class="Ring (严格)"("Disabled"=u8 2) -> ()  [unwired: 2 in, 2 out]
            "CANStartup" <- w743
          }
        }
      }
      event "StartCAN 2": Value Change {
        n718 = event-data() -> ()  [unwired: 7 out]
        n719 = local read "CAN 通道 2"() -> (w744:u32)
        n720 = local read "设备类型"() -> (w749:u32)
        n721 = local read "索引"() -> (w745:u32)
        n722 = dll-call lib="PTH2Kabs J2车用永磁同步电机测试上位机CAN2_源码ControlCAN.dll" fn="VCI_StartCAN"("DeviceType"=w749, "DeviceInd"=w745, "CANInd"=w744) -> (w748:u32)  [unwired: 6 in, 2 out]
        n723 = Equal?(x=w748, y=u32 1) -> (x = y?=w746:bool)
        n724 = case shown="真" w746 {
          selector: w746 -> [_ w751]
          frame False {
          }
          frame True {
            n725 = property on="索引" class="Ring (严格)"("Disabled"=u8 2) -> ()  [unwired: 2 in, 2 out]
            "CANStartup 2" <- w751
          }
        }
      }
      event "ResetCAN": Value Change {
        n726 = event-data() -> ()  [unwired: 7 out]
        n727 = local read "索引"() -> (w758:u32)
        n728 = local read "CAN 通道 2"() -> (w753:u32)
        n729 = local read "设备类型"() -> (w754:u32)
        n730 = dll-call lib="PTH2Kabs J2车用永磁同步电机测试上位机CAN2_源码ControlCAN.dll" fn="VCI_ResetCAN"("DeviceType"=w754, "DeviceInd"=w758, "CANInd"=w753) -> (w755:u32)  [unwired: 6 in, 2 out]
        n731 = local write "CANStartup 2"(FALSE) -> ()
        n732 = Equal?(x=w755, y=u32 1) -> (x = y?=w757:bool)
        n733 = case shown="真" w757 {
          frame False {
          }
          frame True {
            n734 = property on="索引" class="Ring (严格)"("Disabled"=u8 0) -> ()  [unwired: 2 in, 2 out]
          }
        }
      }
      event "Clear Buffer": Value Change {
        (unwired) string[][] [] ("t")
        n735 = event-data() -> ()  [unwired: 2 out]
        n736 = local read "DeviceOpen"() -> (w760:bool)
        n737 = case shown="真" w760 {
          frame False {
          }
          frame True {
            n738 = local read "CAN通道0"() -> (w764:u32)
            n739 = local read "设备类型"() -> (w763:u32)
            n740 = local read "索引"() -> (w762:u32)
            n741 = local read "CAN 通道 2"() -> (w761:u32)
            n742 = dll-call lib="PTH2Kabs J2车用永磁同步电机测试上位机CAN2_源码ControlCAN.dll" fn="VCI_ClearBuffer"("DeviceType"=w763, "DeviceInd"=w762, "CANInd"=w761) -> ()  [unwired: 6 in, 3 out]
            n743 = dll-call lib="PTH2Kabs J2车用永磁同步电机测试上位机CAN2_源码ControlCAN.dll" fn="VCI_ClearBuffer"("DeviceType"=w763, "DeviceInd"=w762, "CANInd"=w764) -> ()  [unwired: 6 in, 3 out]
          }
        }
      }
      event "GetBoardInfo": Value Change {
        n744 = event-data() -> ()  [unwired: 7 out]
        n745 = local read "设备类型"() -> (w767:u32)
        n746 = dll-call lib="PTH2Kabs J2车用永磁同步电机测试上位机CAN2_源码ControlCAN.dll" fn="VCI_ReadBoardInfo"("DeviceType"=u32 0, "DeviceInd"=w767) -> ("VCI_BOARD_INFO"=w765:T5)  [unwired: 5 in, 4 out]
        "VCI_BOARD_INFO" <- w765
        n747 = call "boardinfo.vi"("VCI_BOARD_INFO"=w765) -> ()  [unwired: 1 out]
      }
      event "GetErrorInfo": Value Change {
        n748 = event-data() -> ()  [unwired: 7 out]
        n749 = local read "索引"() -> (w768:u32)
        n750 = local read "CAN通道0"() -> (w770:u32)
        n751 = local read "设备类型"() -> (w771:u32)
        n752 = dll-call lib="PTH2Kabs J2车用永磁同步电机测试上位机CAN2_源码ControlCAN.dll" fn="VCI_ReadErrInfo"("DeviceType"=w771, "DeviceInd"=w768, "CANInd"=w770) -> ("VCI_ERR_INFO"=w769:T6)  [unwired: 6 in, 4 out]
        "VCI_ERR_INFO" <- w769
        n753 = call "errinfo.vi"("VCI_ERR_INFO"=w769) -> ()  [unwired: 1 out]
      }
      event "GetStatus": Value Change {
        n754 = event-data() -> ()  [unwired: 7 out]
        n755 = local read "CAN通道0"() -> (w774:u32)
        n756 = local read "设备类型"() -> (w775:u32)
        n757 = local read "索引"() -> (w772:u32)
        n758 = dll-call lib="PTH2Kabs J2车用永磁同步电机测试上位机CAN2_源码ControlCAN.dll" fn="VCI_ReadCANStatus"("DeviceType"=w775, "DeviceInd"=w772, "CANInd"=w774) -> ("VCI_CAN_STATUS"=w773:T7)  [unwired: 6 in, 4 out]
        "VCI_CAN_STATUS" <- w773
        n759 = call "status.vi"("VCI_CAN_STATUS"=w773) -> ()  [unwired: 1 out]
      }
      event User Event {
        n760 = event-data() -> ("Tx_Or_Rx"=w778:bool, "VCI_CAN_OBJ_N"=w777:T13, "Num"=w776:u32)  [unwired: 2 out]
        n761 = for {
          N: w776 -> [_]
          tunnel: w777 -> [w779] mode=indexing
          tunnel: w778 -> [w789]
          n762 = Unbundle "解除捆绑"(w779) -> ("ID"=w796:u32, "TimeStamp"=w795:u32, "TimeFlag"=w791:u8, "SendType"=w793:u8, "RemoteFlag"=w794:u8, "ExternFlag"=w792:u8, "DataLen"=w790:u8, "Dat1"=w788:u8, "Dat2"=w787:u8, "Dat3"=w786:u8, "Dat4"=w785:u8, "Dat5"=w784:u8, "Dat6"=w783:u8, "Dat7"=w782:u8, "Dat8"=w781:u8)  [unwired: 3 out]
          n763 = Unbundle By Name(w779) -> ("ID"=w780:u32)
          n764 = case shown="102" w780 {
            tunnel: w779 -> [_ w871 w882 w900 w930 w946]
            frame 0, Default {
            }
            frame 256 {
              n765 = Unbundle By Name(w871) -> ("Dat1"=w870:u8, "Dat2"=w869:u8, "Dat3"=w868:u8, "Dat4"=w867:u8, "Dat5"=w865:u8, "Dat6"=w864:u8, "Dat7"=w862:u8, "Dat8"=w861:u8)
              n766 = Join Numbers(hi=w864, lo=w865) -> ((hi.lo)=w863:u16)
              n767 = Join Numbers(hi=w869, lo=w870) -> ((hi.lo)=w856:u16)
              n768 = Join Numbers(hi=w867, lo=w868) -> ((hi.lo)=w866:u16)
              n769 = Join Numbers(hi=w861, lo=w862) -> ((hi.lo)=w860:u16)
              n770 = To Word Integer(number=w856) -> (16bit integer=→"电位器值":i16)
              n771 = To Word Integer(number=w866) -> (16bit integer=→"母线电流零漂":i16)
              n772 = To Word Integer(number=w863) -> (16bit integer=→"U电流零漂":i16)
              n773 = To Word Integer(number=w860) -> (16bit integer=→"V电流零漂":i16)
            }
            frame 257 {
              w873 = 0.1
              n774 = Unbundle By Name(w882) -> ("Dat1"=w888:u8, "Dat2"=w887:u8, "Dat3"=w885:u8, "Dat4"=w886:u8, "Dat5"=w893:u8, "Dat6"=w892:u8, "Dat7"=w884:u8, "Dat8"=w883:u8)
              n775 = Join Numbers(hi=w892, lo=w893) -> ((hi.lo)=w894:u16)
              n776 = Join Numbers(hi=w883, lo=w884) -> ((hi.lo)=w889:u16)
              n777 = Join Numbers(hi=w887, lo=w888) -> ((hi.lo)=w891:u16)
              n778 = Join Numbers(hi=w886, lo=w885) -> ((hi.lo)=w890:u16)
              n779 = To Word Integer(number=w894) -> (16bit integer=w878:i16)
              n780 = To Word Integer(number=w889) -> (16bit integer=w877:i16)
              n781 = To Word Integer(number=w891) -> (16bit integer=w874:i16)
              n782 = To Word Integer(number=w890) -> (16bit integer=w880:i16)
              n783 = Multiply(x=0.01, y=w874) -> (x*y=→"母线电流":dbl)
              n784 = Multiply(x=w873, y=w880) -> (x*y=→"U相电流":dbl)
              n785 = Multiply(x=w873, y=w878) -> (x*y=→"V相电流":dbl)
              n786 = Multiply(x=w873, y=w877) -> (x*y=→"W相电流":dbl)
            }
            frame 258 {
              n787 = Unbundle By Name(w900) -> ("Dat1"=w906:u8, "Dat2"=w905:u8, "Dat3"=w903:u8, "Dat4"=w904:u8, "Dat5"=w910:u8, "Dat6"=w909:u8, "Dat7"=→"系统报警码":u8, "Dat8"=→"控制模式":u8)
              n788 = Join Numbers(hi=w909, lo=w910) -> ((hi.lo)=w911:u16)
              n789 = Join Numbers(hi=w905, lo=w906) -> ((hi.lo)=w908:u16)
              n790 = Join Numbers(hi=w904, lo=w903) -> ((hi.lo)=w907:u16)
              n791 = To Word Integer(number=w907) -> (16bit integer=→"电机转速":i16)
              n792 = To Unsigned Word Integer(number=w908) -> (unsigned 16bit integer=w902:u16)
              n793 = To Unsigned Word Integer(number=w911) -> (unsigned 16bit integer=→"电角度":u16)
              n794 = Multiply(x=0.1, y=w902) -> (x*y=→"母线电压":dbl)
            }
            frame 259 {
              w913 = 0.1
              n795 = Unbundle By Name(w930) -> ("Dat1"=w921:u8, "Dat2"=w920:u8, "Dat3"=w917:u8, "Dat4"=w918:u8, "Dat5"=w935:u8, "Dat6"=w934:u8, "Dat7"=w932:u8, "Dat8"=w931:u8)
              n796 = Join Numbers(hi=w934, lo=w935) -> ((hi.lo)=w936:u16)
              n797 = Join Numbers(hi=w931, lo=w932) -> ((hi.lo)=w933:u16)
              n798 = Join Numbers(hi=w920, lo=w921) -> ((hi.lo)=w919:u16)
              n799 = Join Numbers(hi=w918, lo=w917) -> ((hi.lo)=w915:u16)
              n800 = To Word Integer(number=w919) -> (16bit integer=→"电机扭矩":i16)
              n801 = To Word Integer(number=w933) -> (16bit integer=w929:i16)
              n802 = To Unsigned Word Integer(number=w915) -> (unsigned 16bit integer=w914:u16)
              n803 = To Word Integer(number=w936) -> (16bit integer=w928:i16)
              n804 = Multiply(x=w913, y=w914) -> (x*y=→"VF控制频率":dbl)
              n805 = Multiply(x=w913, y=w928) -> (x*y=w923:dbl)
              "D轴电压Vd" <- w923
              n806 = Multiply(x=w913, y=w929) -> (x*y=w922:dbl)
              "Q轴电压Vq" <- w922
              n807 = Square(x=w923) -> (x^2=w927:dbl)
              n808 = Square(x=w922) -> (x^2=w926:dbl)
              n809 = Add(x=w926, y=w927) -> (x+y=w925:dbl)
              n810 = Square Root(x=w925) -> (sqrt(x)=→"相电压Vs":dbl)
            }
            frame 260 {
              w945 = 0.1
              n811 = Unbundle By Name(w946) -> ("Dat1"=w956:u8, "Dat2"=w955:u8, "Dat3"=w953:u8, "Dat4"=w954:u8, "Dat5"=w961:u8, "Dat6"=w960:u8, "Dat7"=w952:u8, "Dat8"=w951:u8)
              n812 = Join Numbers(hi=w960, lo=w961) -> ((hi.lo)=w962:u16)
              n813 = Join Numbers(hi=w951, lo=w952) -> ((hi.lo)=w957:u16)
              n814 = Join Numbers(hi=w955, lo=w956) -> ((hi.lo)=w959:u16)
              n815 = Join Numbers(hi=w954, lo=w953) -> ((hi.lo)=w958:u16)
              n816 = To Word Integer(number=w958) -> (16bit integer=w949:i16)
              n817 = To Word Integer(number=w957) -> (16bit integer=w948:i16)
              n818 = To Word Integer(number=w959) -> (16bit integer=w950:i16)
              n819 = To Word Integer(number=w962) -> (16bit integer=w947:i16)
              n820 = Multiply(x=w945, y=w949) -> (x*y=w940:dbl)
              "Iq电流指令" <- w940
              n821 = Multiply(x=w945, y=w950) -> (x*y=w939:dbl)
              "Id电流指令" <- w939
              n822 = Multiply(x=w945, y=w947) -> (x*y=→"Id电流":dbl)
              n823 = Multiply(x=w945, y=w948) -> (x*y=→"Iq电流":dbl)
              n824 = Square(x=w939) -> (x^2=w944:dbl)
              n825 = Square(x=w940) -> (x^2=w943:dbl)
              n826 = Add(x=w943, y=w944) -> (x+y=w942:dbl)
              n827 = Square Root(x=w942) -> (sqrt(x)=→"相电流Is":dbl)
            }
          }
          n828 = disable-structure shown="禁用" {
            disable-tunnel: w796 -> [w848 _]
            disable-tunnel: w795 -> [w845 _]
            disable-tunnel: w794 -> [w844 _]
            disable-tunnel: w793 -> [w843 _]
            disable-tunnel: w792 -> [w842 _]
            disable-tunnel: w791 -> [w834 _]
            disable-tunnel: w790 -> [w822 _]
            disable-tunnel: w789 -> [w806 _]
            disable-tunnel: w788 -> [w804 _]
            disable-tunnel: w787 -> [w803 _]
            disable-tunnel: w786 -> [w802 _]
            disable-tunnel: w785 -> [w801 _]
            disable-tunnel: w784 -> [w800 _]
            disable-tunnel: w783 -> [w799 _]
            disable-tunnel: w782 -> [w798 _]
            disable-tunnel: w781 -> [w797 _]
            frame Disabled {
              w833 = 2
              w846 = 8
              n829 = To Unsigned Word Integer() -> ()  [unwired: 1 in, 1 out]
              n830 = local read "TRCount"() -> (w809:u32)
              n831 = Build Array(w804, w803, w802, w801, w800, w799, w798, w797) -> (w823:u8[])
              n832 = Select(t="T", s=w806, f="R") -> (s? t:f=w805:string)
              n833 = Increment(x=w809) -> (x+1=→"TRCount":u32)
              n834 = Number To Hexadecimal String(1:w846, 2:w848) -> (0:w847:string)
              n835 = Number To Decimal String(number=w845, width (-)=w846) -> (decimal integer string=w841:string)
              n836 = Number To Hexadecimal String(1:w833, 2:w834) -> (0:w835:string)
              n837 = Number To Hexadecimal String(1:w833, 2:w843) -> (0:w840:string)
              n838 = Number To Hexadecimal String(1:w833, 2:w844) -> (0:w839:string)
              n839 = Number To Hexadecimal String(1:w833, 2:w842) -> (0:w838:string)
              n840 = Number To Decimal String(number=w822, width (-)=1) -> (decimal integer string=w836:string)
              n841 = Number To Decimal String(number=w809, width (-)=i16 8) -> (decimal integer string=w830:string)
              n842 = for {
                N: w822 -> [_]
                shift-right: [w851] -> w825
                shift-left: "" -> [w849]
                tunnel: w823 -> [w850] mode=indexing
                n843 = Number To Hexadecimal String(1:i16 2 ("width (-)"), 2:w850) -> (0:w853:string)
                n844 = Concatenate Strings(w849, w853, " " ("string")) -> (w851:string)
              }
              n845 = Build Array(w830, w805, w847, w841, w835, w840, w839, w838, w836, w825) -> (w832:string[])
              n846 = local read "Num Rows"() -> (w810:u32)
              n847 = Decrement(x=w810) -> (x-1=w811:u32)
              n848 = Index Array(array=w826, index=0) -> (element=w813)
              n849 = Greater Or Equal?(x=w813, y=1000) -> (x >= y?=w821:bool)
              n850 = Insert Into Array "数组插入"(index (row)=w813, new element=w832) -> (array=w827:string[], w820:string[])  [unwired: 1 in]
              n851 = Array Size(array=w827) -> (size(s)=w826:i32)
              n852 = Select(t=string[][] [], s=w821, f=w820) -> ()  [unwired: 1 out]
              n853 = Greater Or Equal?(x=w813, y=w811) -> (x >= y?=w815:bool)
              n854 = Select(t=w813, s=w815, f=u32 0) -> (s? t:f=w812:u32)
              n855 = Subtract(x=w812, y=w811) -> (x-y=w816:u32)
              n856 = Bundle(w816, u32 0) -> ()  [unwired: 2 out]
            }
            frame Enabled {
            }
          }
        }
      }
      event "确定发送": Value Change {
        n857 = event-data() -> ()  [unwired: 7 out]
        n858 = stacked-sequence {
          frame #0 {
            n859 = case shown="2" "控制模式" {
              selector: "控制模式" -> [w967 w977 w995 w1008]
              frame 0, Default {
                w965 = u8 0
                w970 = u32 0
                n860 = Boolean To (0,1)(Boolean="故障恢复") -> (0, 1=w964:i16)
                n861 = local read "帧格式"() -> (w974:u8)
                n862 = local read "帧类型"() -> (w973:u8)
                n863 = local read "发送类型"() -> (w972:u8)
                n864 = To Unsigned Byte Integer(number=w970) -> (unsigned 8bit integer=w971:u8)
                n865 = Bundle("0x55"=u32 336, w970, w971, "发送类型"=w972, "帧格式"=w974, "帧类型"=w973, 8, "控制模式"=w967, w964, w965, w965, w965, w965, w965, w965, w965, w965, w965) -> (w975:T14)  [unwired: 1 out]
                n866 = local write "VCI_CAN_OBJ_T"(w975) -> ()
              }
              frame 1 {
                w976 = u8 0
                w981 = u32 0
                n867 = local read "帧格式"() -> (w985:u8)
                n868 = local read "帧类型"() -> (w984:u8)
                n869 = local read "发送类型"() -> (w983:u8)
                n870 = To Word Integer(number="给定转速") -> (16bit integer=w989:i16)
                n871 = Split Number(x=w989) -> (hi(x)=w987:u8, lo(x)=w988:u8)
                n872 = To Unsigned Byte Integer(number=w981) -> (unsigned 8bit integer=w982:u8)
                n873 = Bundle("0x55"=u32 336, w981, w982, "发送类型"=w983, "帧格式"=w985, "帧类型"=w984, 8, "控制模式"=w977, u8 1, w988, w987, w976, w976, w976, w976, w976, w976, w976) -> (w986:T15)  [unwired: 1 out]
                n874 = local write "VCI_CAN_OBJ_T"(w986) -> ()
              }
              frame 2 {
                w991 = u8 0
                w999 = u32 0
                n875 = local read "帧格式"() -> (w1003:u8)
                n876 = local read "帧类型"() -> (w1002:u8)
                n877 = local read "发送类型"() -> (w1001:u8)
                n878 = To Word Integer(number="转矩指令") -> (16bit integer=w1005:i16)
                n879 = Split Number(x=w1005) -> (hi(x)=w994:u8, lo(x)=w993:u8)
                n880 = To Unsigned Byte Integer(number=w999) -> (unsigned 8bit integer=w1000:u8)
                n881 = Bundle("0x55"=u32 336, w999, w1000, "发送类型"=w1001, "帧格式"=w1003, "帧类型"=w1002, 8, "控制模式"=w995, u8 1, w991, w991, w993, w994, w991, w991, w991, w991, w991) -> (w1004:T15)  [unwired: 1 out]
                n882 = local write "VCI_CAN_OBJ_T"(w1004) -> ()
              }
              frame 3 {
                w1006 = u8 0
                w1011 = u32 0
                n883 = local read "帧格式"() -> (w1015:u8)
                n884 = local read "帧类型"() -> (w1014:u8)
                n885 = local read "发送类型"() -> (w1013:u8)
                n886 = To Unsigned Byte Integer(number=w1011) -> (unsigned 8bit integer=w1012:u8)
                n887 = Bundle("0x55"=u32 336, w1011, w1012, "发送类型"=w1013, "帧格式"=w1015, "帧类型"=w1014, 8, "控制模式"=w1008, u8 1, w1006, w1006, w1006, w1006, w1006, w1006, w1006, w1006, w1006) -> (w1016:T15)  [unwired: 1 out]
                n888 = local write "VCI_CAN_OBJ_T"(w1016) -> ()
              }
            }
          }
        }
      }
      event "确定发送 2": Value Change {
        n889 = event-data() -> ()  [unwired: 7 out]
      }
      event "增加": Value Change {
        n890 = event-data() -> ()  [unwired: 7 out]
        n891 = case shown="真" "增加" {
          frame False {
          }
          frame True {
            n892 = local read "给定转速"() -> (w1019:dbl)
            n893 = local read "转速梯度"() -> (w1018:dbl)
            n894 = Add(x=w1019, y=w1018) -> (x+y=w1020:dbl)
            n895 = local write "给定转速"(w1020) -> ()
          }
        }
      }
      event "增加 2": Value Change {
        n896 = event-data() -> ()  [unwired: 7 out]
        n897 = case shown="真" "增加 2" {
          frame False {
          }
          frame True {
            n898 = local read "转矩指令"() -> (w1023:dbl)
            n899 = local read "扭矩梯度"() -> (w1022:dbl)
            n900 = Add(x=w1023, y=w1022) -> (x+y=w1024:dbl)
            n901 = local write "转矩指令"(w1024) -> ()
          }
        }
      }
      event "减少": Value Change {
        n902 = event-data() -> ()  [unwired: 7 out]
        n903 = case shown="真" "减少" {
          frame False {
          }
          frame True {
            n904 = local read "给定转速"() -> (w1027:dbl)
            n905 = local read "转速梯度"() -> (w1028:dbl)
            n906 = Subtract(x=w1027, y=w1028) -> (x-y=w1026:dbl)
            n907 = local write "给定转速"(w1026) -> ()
          }
        }
      }
      event "减少 2": Value Change {
        n908 = event-data() -> ()  [unwired: 7 out]
        n909 = case shown="真" "减少 2" {
          frame False {
          }
          frame True {
            n910 = local read "转矩指令"() -> (w1032:dbl)
            n911 = local read "扭矩梯度"() -> (w1031:dbl)
            n912 = Subtract(x=w1032, y=w1031) -> (x-y=w1030:dbl)
            n913 = local write "转矩指令"(w1030) -> ()
          }
        }
      }
      event "SEND_NCAN": Value Change {
        n914 = event-data() -> ()  [unwired: 7 out]
        n915 = case shown="真" "SEND_NCAN" {
          frame False {
          }
          frame True {
            n916 = stacked-sequence {
              frame #0 {
                n917 = local read "VCI_CAN_OBJ_T"() -> (w1035:T8)
                n918 = Build Array(w1035, w1035, w1035, w1035, w1035, w1035, w1035, w1035, w1035, w1035, w1035, w1035, w1035) -> (w1034:T4)
                n919 = local write "VCI_CAN_OBJ_T_N"(w1034) -> ()
              }
              frame #1 {
                n920 = local read "VCI_CAN_OBJ_T_N"() -> (w1040:T4)
                n921 = local read "索引"() -> (w1036:u32)
                n922 = local read "CAN通道0"() -> (w1042:u32)
                n923 = local read "设备类型"() -> (w1041:u32)
                n924 = dll-call lib="PTH2Kabs J2车用永磁同步电机测试上位机CAN2_源码ControlCAN.dll" fn="VCI_Transmit"("DeviceType"=w1041, "DeviceInd"=w1036, "CANInd"=w1042, "pSend"=w1040, "Len"=u32 13) -> ("返回类型"=w1038:u32)  [unwired: 8 in, 2 out]
                n925 = Equal?(x=w1038, y=u32 13) -> (x = y?=w1037:bool)
                n926 = case shown="真" w1037 {
                  frame False {
                    n927 = call "显示对话框信息2"() -> ()  [unwired: 3 in, 9 out]
                  }
                  frame True {
                    n928 = call "显示对话框信息"() -> ()  [unwired: 3 in, 9 out]
                  }
                }
              }
            }
          }
        }
      }
    }
  }
  n929 = while {
    tunnel: w3 -> [w1049]
    tunnel: w2 -> [w1048]
    tunnel: [w1047] -> _
    tunnel: [w1046] -> _
    stop <- w1044 stop-if-true
    n930 = local read "CANStartup"() -> (w1045:bool)
    n931 = case shown="真" w1045 {
      tunnel: w1049 -> [w1052 w1066]
      tunnel: w1048 -> [w1051 w1065]
      tunnel: [w1052 w1064] -> w1047
      tunnel: [w1051 w1063] -> w1046
      frame False {
        n932 = Wait Until Next ms Multiple(millisecond multiple=u32 10) -> ()  [unwired: 1 out]
      }
      frame True {
        n933 = local read "CAN通道0"() -> (w1059:u32)
        n934 = local read "设备类型"() -> (w1061:u32)
        n935 = local read "索引"() -> (w1060:u32)
        n936 = dll-call lib="PTH2Kabs J2车用永磁同步电机测试上位机CAN2_源码ControlCAN.dll" fn="VCI_GetReceiveNum"("DeviceType"=w1061, "DeviceInd"=w1060, "CANInd"=w1059) -> ("return type"=w1053:u32)  [unwired: 6 in, 2 out]
        n937 = Greater Or Equal?(x=w1053, y=u32 1) -> (x >= y?=w1054:bool)
        n938 = case shown="真" w1054 {
          tunnel: [_ w1070] -> w1058
          tunnel: [_ w1069] -> w1057
          tunnel: [_ w1068] -> w1056
          tunnel: w1053 -> [_ w1067]
          frame False {
          }
          frame True {
            n939 = local read "VCI_CAN_OBJ_RN"() -> (w1074:T4)
            n940 = local read "CAN通道0"() -> (w1072:u32)
            n941 = local read "设备类型"() -> (w1073:u32)
            n942 = local read "索引"() -> (w1076:u32)
            n943 = dll-call lib="PTH2Kabs J2车用永磁同步电机测试上位机CAN2_源码ControlCAN.dll" fn="VCI_Receive"("DeviceType"=w1073, "DeviceInd"=w1076, "CANInd"=w1072, "pReceive"=w1074, "Len"=w1067, "WaitTime"=100) -> ("return type"=w1070:u32, "pReceive"=w1068:T4)  [unwired: 8 in, 2 out]
            n944 = local write "VCI_CAN_OBJ_RN"(w1068) -> ()
            n945 = Greater Or Equal?(x=w1070, y=u32 1) -> (x >= y?=w1069:bool)
          }
        }
        n946 = local read "VCI_CAN_OBJ_R"() -> (w1062:T8)
        n947 = case shown="真" w1057 {
          tunnel: w1066 -> [w1078 w1087]
          tunnel: w1065 -> [w1077 w1086]
          tunnel: [w1078 w1085] -> w1064
          tunnel: [w1077 w1084] -> w1063
          tunnel: w1056 -> [_ w1081]
          tunnel: w1058 -> [_ w1080]
          tunnel: w1062 -> [_ w1079]
          frame False {
          }
          frame True {
            n948 = Bundle(FALSE, "VCI_CAN_OBJ_R"=w1079, "pReceive"=w1081, "return type"=w1080) -> (w1082:T16)  [unwired: 1 out]
            n949 = Generate User Event "产生用户事件"(user event=w1087, event data cluster=w1082, error in=w1086) -> (user event out=w1085:refnum<user-event>, error out=w1084:errorcluster)  [unwired: 1 in]
          }
        }
      }
    }
    n950 = local read "stop 2"() -> (w1044:bool)
  }
  n951 = local read "设备类型"() -> (w12:u32)
  n952 = Equal?(x=w12, y=w16) -> (x = y?=w11:bool)
  n953 = Equal?(x=w12, y=w15) -> (x = y?=w10:bool)
  n954 = Equal?(x=w12, y=w14) -> (x = y?=w9:bool)
  n955 = Equal?(x=w12, y=w13) -> (x = y?=w8:bool)
  n956 = Or(x=w9, y=w8) -> (x .or. y?=w6:bool)
  n957 = Or(x=w11, y=w10) -> (x .or. y?=w7:bool)
  n958 = Or(x=w7, y=w6) -> (x .or. y?=w5:bool)
  n959 = case shown="假" w5 {
    frame False {
      n960 = stacked-sequence {
        frame #0 {
          n961 = local write "Radio_Baud"(FALSE) -> ()
        }
        frame #1 {
          n962 = local read "Baud"() -> (w1089:u32)
          n963 = case shown="1" w1089 {
            frame 0 {
              n964 = local write "BTR0"(u8 191 ("BTR0")) -> ()
              n965 = local write "BTR1"(u8 255 ("BTR1")) -> ()
            }
            frame 1 {
              n966 = local write "BTR0"(u8 49 ("BTR0")) -> ()
              n967 = local write "BTR1"(u8 28 ("BTR1")) -> ()
            }
            frame 2 {
              n968 = local write "BTR0"(u8 24 ("BTR0")) -> ()
              n969 = local write "BTR1"(u8 28 ("BTR1")) -> ()
            }
            frame 3 {
              n970 = local write "BTR1"(u8 255 ("BTR1")) -> ()
              n971 = local write "BTR0"(u8 135 ("BTR0")) -> ()
            }
            frame 4 {
              n972 = local write "BTR1"(u8 28 ("BTR1")) -> ()
              n973 = local write "BTR0"(u8 9 ("BTR0")) -> ()
            }
            frame 5 {
              n974 = local write "BTR0"(u8 131 ("BTR0")) -> ()
              n975 = local write "BTR1"(u8 255 ("BTR1")) -> ()
            }
            frame 6 {
              n976 = local write "BTR1"(u8 28 ("BTR1")) -> ()
              n977 = local write "BTR0"(u8 4 ("BTR0")) -> ()
            }
            frame 7 {
              n978 = local write "BTR0"(u8 3 ("BTR0")) -> ()
              n979 = local write "BTR1"(u8 28 ("BTR1")) -> ()
            }
            frame 8 {
              n980 = local write "BTR0"(u8 129 ("BTR0")) -> ()
              n981 = local write "BTR1"(u8 250 ("BTR1")) -> ()
            }
            frame 9 {
              n982 = local write "BTR1"(u8 28 ("BTR1")) -> ()
              n983 = local write "BTR0"(u8 1 ("BTR0")) -> ()
            }
            frame 10 {
              n984 = local write "BTR0"(u8 128 ("BTR0")) -> ()
              n985 = local write "BTR1"(u8 250 ("BTR1")) -> ()
            }
            frame 11 {
              n986 = local write "BTR0"(u8 0 ("BTR0")) -> ()
              n987 = local write "BTR1"(u8 28 ("BTR1")) -> ()
            }
            frame 12 {
              n988 = local write "BTR0"(u8 128 ("BTR0")) -> ()
              n989 = local write "BTR1"(u8 182 ("BTR1")) -> ()
            }
            frame 13 {
              n990 = local write "BTR1"(u8 22 ("BTR1")) -> ()
              n991 = local write "BTR0"(u8 0 ("BTR0")) -> ()
            }
            frame 14 {
              n992 = local write "BTR0"(u8 0 ("BTR0")) -> ()
              n993 = local write "BTR1"(u8 20 ("BTR1")) -> ()
            }
            frame 15, Default {
            }
          }
        }
      }
    }
    frame True {
      n994 = stacked-sequence {
        frame #0 {
          n995 = local write "Radio_Baud(E_U)"(FALSE) -> ()
          n996 = local write "BTR1"(u8 0 ("BTR1")) -> ()
          n997 = local write "BTR0"(u8 0 ("BTR0")) -> ()
        }
        frame #1 {
          n998 = local read "Baud"() -> (w1123:u32)
          n999 = case shown="15, 默认" w1123 {
            frame 15, Default {
            }
            frame 14 {
              n1000 = local write "寄存器"(393219) -> ()
            }
            frame 13 {
              n1001 = local write "寄存器"(393220) -> ()
            }
            frame 11 {
              n1002 = local write "寄存器"(393223) -> ()
            }
            frame 9 {
              n1003 = local write "寄存器"(1835016) -> ()
            }
            frame 7 {
              n1004 = local write "寄存器"(1835025) -> ()
            }
            frame 6 {
              n1005 = local write "寄存器"(1441827) -> ()
            }
            frame 4 {
              n1006 = local write "寄存器"(1835052) -> ()
            }
            frame 2 {
              n1007 = local write "寄存器"(1441971) -> ()
            }
            frame 1 {
              n1008 = local write "寄存器"(1835232) -> ()
            }
            frame 0 {
              n1009 = local write "寄存器"(1835457) -> ()
            }
          }
        }
      }
    }
  }
  n1010 = local write "CANET IP"("192.168.21.78" ("CANET IP")) -> ()
  n1011 = while {
    tunnel: w3 -> [w1139]
    tunnel: w2 -> [w1138]
    tunnel: [w1137] -> _
    tunnel: [w1136] -> _
    stop <- w1135 stop-if-true
    n1012 = local read "CANStartup 2"() -> (w1134:bool)
    n1013 = case shown="真" w1134 {
      tunnel: w1139 -> [w1142 w1156]
      tunnel: w1138 -> [w1141 w1155]
      tunnel: [w1142 w1154] -> w1137
      tunnel: [w1141 w1153] -> w1136
      frame False {
        n1014 = Wait Until Next ms Multiple(millisecond multiple=u32 10) -> ()  [unwired: 1 out]
      }
      frame True {
        n1015 = local read "CAN 通道 2"() -> (w1143:u32)
        n1016 = local read "设备类型"() -> (w1151:u32)
        n1017 = local read "索引"() -> (w1150:u32)
        n1018 = dll-call lib="PTH2Kabs J2车用永磁同步电机测试上位机CAN2_源码ControlCAN.dll" fn="VCI_GetReceiveNum"("DeviceType"=w1151, "DeviceInd"=w1150, "CANInd"=w1143) -> ("return type"=w1144:u32)  [unwired: 6 in, 2 out]
        n1019 = Greater Or Equal?(x=w1144, y=u32 1) -> (x >= y?=w1145:bool)
        n1020 = case shown="真" w1145 {
          tunnel: [_ w1162] -> w1149
          tunnel: [_ w1161] -> w1148
          tunnel: [_ w1160] -> w1147
          tunnel: w1144 -> [_ w1159]
          frame False {
          }
          frame True {
            n1021 = local read "CAN 通道 2"() -> (w1157:u32)
            n1022 = local read "VCI_CAN_OBJ_RN"() -> (w1164:T4)
            n1023 = local read "设备类型"() -> (w1158:u32)
            n1024 = local read "索引"() -> (w1166:u32)
            n1025 = dll-call lib="PTH2Kabs J2车用永磁同步电机测试上位机CAN2_源码ControlCAN.dll" fn="VCI_Receive"("DeviceType"=w1158, "DeviceInd"=w1166, "CANInd"=w1157, "pReceive"=w1164, "Len"=w1159, "WaitTime"=100) -> ("return type"=w1162:u32, "pReceive"=w1160:T4)  [unwired: 8 in, 2 out]
            n1026 = local write "VCI_CAN_OBJ_RN"(w1160) -> ()
            n1027 = Greater Or Equal?(x=w1162, y=u32 1) -> (x >= y?=w1161:bool)
          }
        }
        n1028 = local read "VCI_CAN_OBJ_R"() -> (w1152:T8)
        n1029 = case shown="真" w1148 {
          tunnel: w1156 -> [w1168 w1177]
          tunnel: w1155 -> [w1167 w1176]
          tunnel: [w1168 w1175] -> w1154
          tunnel: [w1167 w1174] -> w1153
          tunnel: w1147 -> [_ w1171]
          tunnel: w1149 -> [_ w1170]
          tunnel: w1152 -> [_ w1169]
          frame False {
          }
          frame True {
            n1030 = Bundle(FALSE, "VCI_CAN_OBJ_R"=w1169, "pReceive"=w1171, "return type"=w1170) -> (w1172:T16)  [unwired: 1 out]
            n1031 = Generate User Event "产生用户事件"(user event=w1177, event data cluster=w1172, error in=w1176) -> (user event out=w1175:refnum<user-event>, error out=w1174:errorcluster)  [unwired: 1 in]
          }
        }
      }
    }
    n1032 = local read "stop 2"() -> (w1135:bool)
  }
  n1033 = local write "CANET 端口"(u32 4002 ("CANET 端口")) -> ()
  n1034 = local write "本机端口"(u32 4003 ("本机端口")) -> ()
  n1035 = while {
    tunnel: w3 -> [w1183]
    tunnel: w2 -> [w1182]
    tunnel: [w1185] -> w33
    tunnel: [w1184] -> w32
    stop <- w1181 stop-if-true
    n1036 = Or(x="确定发送", y="确定发送 2") -> (x .or. y?=w1179:bool)
    n1037 = case shown="假" w1179 {
      tunnel: [w1187 w1199] -> w1185
      tunnel: [w1188 w1198] -> w1184
      tunnel: w1183 -> [w1188 w1197]
      tunnel: w1182 -> [w1187 w1196]
      tunnel: "确定发送" -> [_ w1190]
      frame False {
        n1038 = Wait Until Next ms Multiple(millisecond multiple=u32 10) -> ()  [unwired: 1 out]
      }
      frame True {
        n1039 = case shown="假" w1190 {
          tunnel: [w1203 w1204] -> w1189
          frame False {
            n1040 = local read "CAN 通道 2"() -> (w1203:u32)
          }
          frame True {
            n1041 = local read "CAN通道0"() -> (w1204:u32)
          }
        }
        n1042 = local read "一次发送帧数"() -> (w1195:u32)
        n1043 = local read "设备类型"() -> (w1202:u32)
        n1044 = local read "索引"() -> (w1191:u32)
        n1045 = for {
          N: w1195 -> [_]
          tunnel: [w1205] -> w1193 mode=indexing
          tunnel: [w1205] -> w1192
          n1046 = local read "VCI_CAN_OBJ_T"() -> (w1205:T8)
        }
        n1047 = dll-call lib="PTH2Kabs J2车用永磁同步电机测试上位机CAN2_源码ControlCAN.dll" fn="VCI_Transmit"("DeviceType"=w1202, "DeviceInd"=w1191, "CANInd"=w1189, "pSend"=w1193, "Len"=w1195) -> ("return type"=w1194:u32)  [unwired: 7 in, 3 out]
        n1048 = Greater Or Equal?(x=w1194, y=u32 1) -> (x >= y?=w1200:bool)
        n1049 = local write "VCI_CAN_OBJ_TN"(w1193) -> ()
        n1050 = case shown="真" w1200 {
          tunnel: w1197 -> [w1207 w1216]
          tunnel: w1196 -> [w1206 w1215]
          tunnel: [w1206 w1214] -> w1199
          tunnel: [w1207 w1213] -> w1198
          tunnel: w1194 -> [_ w1210]
          tunnel: w1193 -> [_ w1209]
          tunnel: w1192 -> [_ w1208]
          frame False {
            n1051 = call "Display Message to User"() -> ()  [unwired: 3 in, 9 out]
          }
          frame True {
            n1052 = Bundle(TRUE, "VCI_CAN_OBJ_T"=w1208, w1209, "return type"=w1210) -> (w1211:T17)  [unwired: 1 out]
            n1053 = Generate User Event(user event=w1216, event data cluster=w1211, error in=w1215) -> (user event out=w1213:refnum<user-event>, error out=w1214:errorcluster)  [unwired: 1 in]
          }
        }
      }
    }
    n1054 = local read "stop 2"() -> (w1181:bool)
  }
  n1055 = while {
    stop <- w1218 stop-if-true
    n1056 = case shown="真" "自动记录 2" {
      frame False {
        n1057 = local write "记录计数 3"(0) -> ()
      }
      frame True {
        n1058 = stacked-sequence {
          seq-local: [w1222 _ _] -> [_ w1260 w1263]
          seq-local: [_ w1257 _] -> [_ _ w1264]
          frame #0 {
            n1059 = local read "记录计数 3"() -> (w1222:u32)
            n1060 = Equal To 0?(x=w1222) -> (x = 0?=w1221:bool)
            n1061 = case shown="真" w1221 {
              frame False {
              }
              frame True {
                w1233 = "Num,Time,转速指令,母线电流偏执,U相电流偏执,V相电流偏执,转矩指令,U相电流,V相电流,W相电流,母线电压,电机转速,电角度位置,控制模式,相电流Is,相电压Vs,D轴电压,Q轴电压,D轴电流指令,Q轴电流指令,D轴电流,Q轴电流,电机扭矩,系统报警码\n "  # Num,Time,转速指令,母线电流偏执,U相电流偏执,V相电流偏执,转矩指令,U相电流,V相电流,W相电流,母线电压,电机转速,电角度位置,控制模式,相电流Is,相电压Vs,D轴电压,Q轴电压,D轴电流指令,Q轴电流指令,D轴电流,Q轴电流,电机扭矩,系统报警码
                n1062 = local read "保存路径 2"() -> (w1223:path)
                n1063 = Open/Create/Replace File(file path (use dialog)=w1223, operation (0:open)=3, access (0:read/write)=0) -> (refnum out=w1230:refnum<file>, error out=w1229:errorcluster)  [unwired: 3 in, 1 out]
                n1064 = Set File Position(refnum=w1230, from (0:start)=enum16{"start", "end", "current"}."end" ("自（0:起始）"), error in=w1229) -> (refnum out=w1231:refnum<file>, error out=w1228:errorcluster)  [unwired: 1 in]
                n1065 = Write to Text File(file (use dialog)=w1231, text=w1233, error in=w1228) -> (refnum out=w1227:refnum<file>, error out=w1226:errorcluster)  [unwired: 1 in, 1 out]
                n1066 = Close File(refnum=w1227, error in=w1226) -> ()  [unwired: 2 out]
              }
            }
          }
          frame #1 {
            n1067 = local read "母线电流零漂"() -> (w1254:u16)
            n1068 = local read "U电流零漂"() -> (w1253:u16)
            n1069 = local read "Q轴电压Vq"() -> (w1251:dbl)
            n1070 = local read "相电压Vs"() -> (w1242:dbl)
            n1071 = local read "V电流零漂"() -> (w1252:u16)
            n1072 = local read "电机转速"() -> (w1247:dbl)
            n1073 = local read "母线电压"() -> (w1246:dbl)
            n1074 = local read "相电流Is"() -> (w1243:dbl)
            n1075 = local read "W相电流"() -> (w1248:dbl)
            n1076 = local read "控制模式"() -> (w1244:u8)
            n1077 = local read "电角度"() -> (w1245:u16)
            n1078 = local read "电位器值"() -> (w1255:i16)
            n1079 = local read "V相电流"() -> (w1249:dbl)
            n1080 = local read "U相电流"() -> (w1250:dbl)
            n1081 = Format Date/Time String(time format string (%c)="%#H:%#M:%#S") -> (date/time string=w1258:string)  [unwired: 2 in]
            n1082 = local read "系统报警码"() -> (w1234:u16)
            n1083 = local read "D轴电压Vd"() -> (w1241:dbl)
            n1084 = local read "Q轴电压Vq"() -> (w1240:dbl)
            n1085 = local read "Iq电流指令"() -> (w1238:dbl)
            n1086 = local read "Id电流指令"() -> (w1239:dbl)
            n1087 = local read "电机扭矩"() -> (w1235:dbl)
            n1088 = local read "Id电流"() -> (w1237:dbl)
            n1089 = local read "Iq电流"() -> (w1236:dbl)
            n1090 = Format Into String(format string="%d,%s,%d,%d,%d,%d,%f,%f,%f,%f,%f,%d,%d,%d,%f,%f,%f,%f,%f,%f,%f,%f,%d,%d\\n", w1260, w1258, w1255, w1254, w1253, w1252, w1251, w1250, w1249, w1248, w1246, w1247, w1245, w1244, w1243, w1242, w1241, w1240, w1239, w1238, w1237, w1236, w1235, w1234) -> (resulting string=w1257:string)  [unwired: 2 in, 1 out]
          }
          frame #2 {
            n1091 = Increment(x=w1263) -> (x+1=w1262:u32)
            n1092 = local write "记录计数 3"(w1262) -> ()
            n1093 = Open/Create/Replace File(file path (use dialog)="保存路径 2", operation (0:open)=3, access (0:read/write)=0) -> (refnum out=w1271:refnum<file>, error out=w1273:errorcluster)  [unwired: 3 in, 1 out]
            n1094 = Set File Position(refnum=w1271, from (0:start)=1, error in=w1273) -> (refnum out=w1268:refnum<file>, error out=w1269:errorcluster)  [unwired: 1 in]
            n1095 = Write to Text File(file (use dialog)=w1268, text=w1264, error in=w1269) -> (refnum out=w1266:refnum<file>, error out=w1267:errorcluster)  [unwired: 1 in, 1 out]
            n1096 = Close File(refnum=w1266, error in=w1267) -> ()  [unwired: 2 out]
          }
        }
      }
    }
    n1097 = Wait Until Next ms Multiple(millisecond multiple=u32 10 ("周期")) -> ()  [unwired: 1 out]
    n1098 = local read "stop 2"() -> (w1218:bool)
  }
  n1099 = while {
    stop <- w1276 stop-if-true
    n1100 = case shown="真" "打开曲线" {
      frame False {
      }
      frame True {
        n1101 = local read "Id电流指令"() -> (w1282:dbl)
        n1102 = local read "Iq电流指令"() -> (w1281:dbl)
        n1103 = local read "D轴电压Vd"() -> (w1278:dbl)
        n1104 = local read "Q轴电压Vq"() -> (w1277:dbl)
        n1105 = local read "电机扭矩"() -> (w1283:dbl)
        n1106 = local read "电机转速"() -> (w1284:dbl)
        n1107 = local read "Id电流"() -> (w1280:dbl)
        n1108 = local read "Iq电流"() -> (w1279:dbl)
        n1109 = Bundle("电机转速"=w1284, "电机扭矩"=w1283, "Id电流指令"=w1282, "Iq电流指令"=w1281, "Id电流"=w1280, "Iq电流"=w1279, "D轴电压Vd"=w1278, "Q轴电压Vq"=w1277) -> (→"波形图表":T18)  [unwired: 1 in]
      }
    }
    n1110 = Wait Until Next ms Multiple(millisecond multiple=u32 10 ("周期")) -> ()  [unwired: 1 out]
    n1111 = local read "stop 2"() -> (w1276:bool)
  }
  n1112 = Unregister For Events "取消注册事件"(event registration refnum=w1, error in=w33) -> (error out=w36:errorcluster)
  n1113 = local write "CANStartup"(w4) -> ()
  n1114 = local write "TRCount"(u32 0 ("TRCount")) -> ()
  n1115 = local write "CANStartup 2"(w4) -> ()
  n1116 = local write "stop 2"(FALSE ("stop 2")) -> ()
  n1117 = Destroy User Event "销毁用户事件"(user event=w32, error in=w36) -> ()  [unwired: 1 out]
  "type" <- u8[] [1, 0, 0, 0] ("type")
